vi "Autonomous Independent.vi"() -> ()   [LabVIEW 2015]
doc: "This VI is called when autonomous begins, and will automatically be terminated when autonomous ends. You can carry out timed or sensor driven robot movement independently without needing to return to the caller."
uses:
  <vilib>/Rock Robotics/WPI/DriverStation/WPI_DriverStationMatch Info.ctl
  <vilib>/Rock Robotics/WPI/Utilities/WPI_GetSetVariantRefNum.vi
  <vilib>/Rock Robotics/Network Tables/NT Write Numeric Array.vi
  <vilib>/Rock Robotics/Network Tables/NT Read String.vi
  <vilib>/Rock Robotics/WPI/Solenoid/Deprecated/WPI_SolenoidSetBool.vi
  <vilib>/Rock Robotics/WPI/RobotDrive/WPI_RobotDriveArcadeDrive_Standard(NoSaturation).vi
  Global 1.vi
  Global 2.vi
  <vilib>/functionblocks/Counter/Pulse Timer/Pulse Timer.vi
  <vilib>/functionblocks/Counter/Timer On Delay/Timer On Delay.vi
  <vilib>/Rock Robotics/Network Tables/NT Write Boolean.vi
  <vilib>/functionblocks/FB Core/FB Core.xnode
  <vilib>/Rock Robotics/WPI/SafetyOutput/WPI_SafetyOutputConfigMenu.ctl
  <vilib>/functionblocks/NI_FunctionBlock Libraries.lvlib
panel:
  out "Actual Arm Angle":dbl
  out "Arm Speed":dbl
  out "Arm Request":dbl
  out "Vert Gyro Angle":dbl
  out "Horz Gyro Angle":dbl
  out "Position":string
  out "Defense":string
  out "Right Distance":dbl
  out "Left Distance":dbl
  in  "Match Info":T1={"Autonomous Elapsed Seconds"=0.0, "TeleOp Elapsed Seconds"=0.0, "Disabled Elapsed Seconds"=0.0, "Visited Autonomous"=FALSE, "Visited TeleOp"=FALSE, "Visited Disabled"=FALSE, "Autonomous Settings"={"Autonomous Style"=enum."Independent", "VI Refnum"=refnum}}
  out "Current Movement, for debugging":T2 {"Y Joystick Value" scale=1.0..-1.0; "X Joystick Value" scale=-1.0..1.0}
  in  "Array of robot movements":T3(array[cluster])=[{"X Joystick Value"=0.39393939393939403, "Y Joystick Value"=0.0, "Delay (sec)"=1.0, "Movement Name"="turn"}, {"X Joystick Value"=-0.3737373737373737, "Y Joystick Value"=0.0, "Delay (sec)"=1.0, "Movement Name"="turn back"}] {"Y Joystick Value" scale=1.0..-1.0; "X Joystick Value" scale=-1.0..1.0}
  # "Be sure to right-click and choose Data Operations>>Make Current Value default if you want to save the array values with the VI"
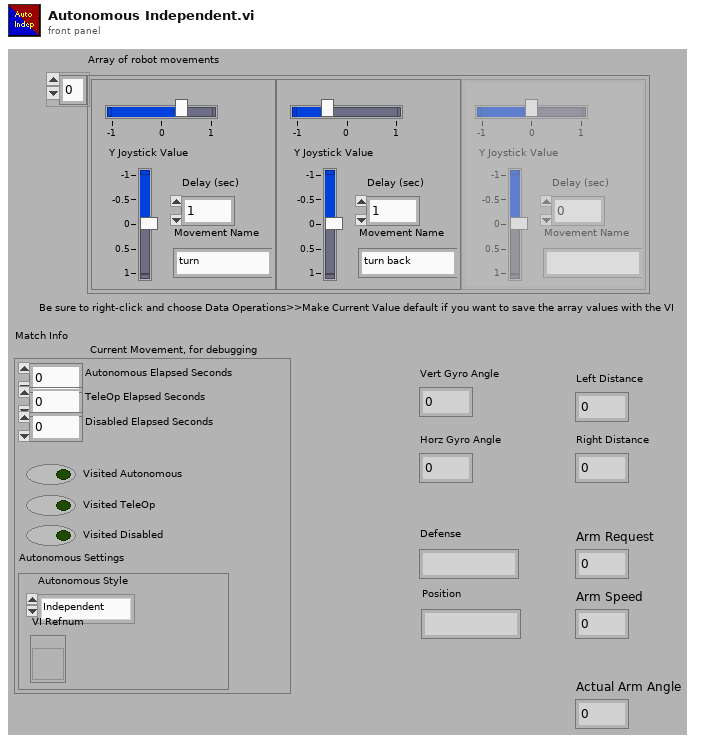
[diagram p1: front panel]
types:
  T1 = typedef "WPI_DriverStationMatch Info.ctl" = cluster{"Autonomous Elapsed Seconds":dbl, "TeleOp Elapsed Seconds":dbl, "Disabled Elapsed Seconds":dbl, "Visited Autonomous":bool, "Visited TeleOp":bool, "Visited Disabled":bool, "Autonomous Settings":cluster{"Autonomous Style":enum16{"Iterative", "Independent"}, "VI Refnum":refnum<vi>}}
  T2 = cluster{"X Joystick Value":dbl, "Y Joystick Value":dbl, "Delay (sec)":dbl, "Movement Name":string}
  T3 = cluster{"X Joystick Value":dbl, "Y Joystick Value":dbl, "Delay (sec)":dbl, "Movement Name":string}[]
  T4 = typedef "WPI_GyroDevRef.ctl" = cluster{"DevStatus":errorcluster, "Analog Channel":T5, "Offset":dbl, "Gain (VoltsPerDegree/Second)":dbl, "Gyro Type":enum16{"Analog", "XRS450"}, "Handle":i32, "SPI Bus":T6, "Device Found":bool, "Sample Rate":dbl, "Calibrate On Open":bool}
  T5 = typedef "FPGA_AIChannel.ctl" = enum8{"AI 0", "AI 1", "AI 2", "AI 3", "AI MXP 0", "AI MXP 1", "AI MXP 2", "AI MXP 3", "Invalid"}
  T6 = typedef "spi_bus.ctl" = enum16{"SPI On-Board, CS0", "SPI On-Board, CS1", "SPI On-Board, CS2", "SPI On-Board, CS3", "SPI MXP", "Invalid"}
  T7 = typedef "WPI_EncoderDevRef.ctl" = cluster{"DevStatus":errorcluster, "EncoderIndex":T8, "CounterIndex":T9, "DistancePerCount":dbl, "Decoding Type":T10}
  T8 = typedef "FPGA_EncoderIdx.ctl" = enum8{"Enc 0", "Enc 1", "Enc 2", "Enc 3", "Enc 4", "Enc 5", "Enc 6", "Enc 7", "Invalid"}
  T9 = typedef "FPGA_CounterCtrSystemIndex.ctl" = enum8{"Ctr 0", "Ctr 1", "Ctr 2", "Ctr 3", "Ctr 4", "Ctr 5", "Ctr 6", "Ctr 7", "Invalid"}
  T10 = typedef "WPI_EncoderType.ctl" = enum16{"1x", "2x", "4x"}
  T11 = typedef "WPI_JoystickDevRef.ctl" = cluster{"Device":T12}
  T12 = typedef "WPI_JoystickDeviceEnum.ctl" = enum16{"USB 0", "USB 1", "USB 2", "USB 3", "USB 4", "USB 5"}
  T13 = typedef "WPI_PotentiometerDevRef.ctl" = cluster{"DevStatus":errorcluster, "Analog Channel":T5, "Invert Output":bool}
  T14 = typedef "WPI_SolenoidDevRef.ctl" = cluster{"DevStatus":errorcluster, "Pneumatics Control Module":u8, "Forward Solenoid Channel":T15, "Reverse Solenoid Channel":T15}
  T15 = typedef "WPI_SolenoidChannel.ctl" = enum8{"Solenoid 0", "Solenoid 1", "Solenoid 2", "Solenoid 3", "Solenoid 4", "Solenoid 5", "Solenoid 6", "Solenoid 7", "Invalid"}
  T16 = typedef "WPI_RobotDriveDevRef.ctl" = cluster{"DevStatus":errorcluster, "Motors[]":T17[], "Square Inputs":bool, "Max Output":dbl}
  T17 = typedef "WPI_MotorControlDeviceRef.ctl" = cluster{"DeviceStatus":errorcluster, "Type":T18, "PWM":cluster{"PWM Channel":T19, "DeadBand":T20}, "CAN":cluster{"Device Number":u8, "Control Mode":T21, "Semaphore":T22, "Max Vout":dbl, "TalonSRX Control Mode":T23}, "Invert":bool}
  T18 = typedef "WPI_MotorControlType.ctl" = enum16{"PWM", "CAN", "CANTalonSRX"}
  T19 = typedef "FPGA_DIOPWMChannel.ctl" = enum8{"PWM 0", "PWM 1", "PWM 2", "PWM 3", "PWM 4", "PWM 5", "PWM 6", "PWM 7", "PWM 8", "PWM 9", "PWM MXP 0", "PWM MXP 1", "PWM MXP 2", "PWM MXP 3", "PWM MXP 4", "PWM MXP 5", "PWM MXP 6", "PWM MXP 7", "PWM MXP 8", "PWM MXP 9", "Invalid"}
  T20 = typedef "WPI_PWMDeadband.ctl" = cluster{"Name":string, "maxPositivePwm":i32, "minPositivePwm":i32, "centerPwm":i32, "maxNegativePwm":i32, "minNegativePwm":i32, "angularRange":u16}
  T21 = typedef "WPI_CANJaguar_ControlMode.ctl" = enum8{"Percent VBus", "Current", "Speed", "Position", "Voltage"}
  T22 = typedef "Semaphore RefNum" = refnum<k1>
  T23 = typedef "WPI_CANTalonSRX_APIControlMode.ctl" = enum8{"Percent VBus", "Speed", "Position", "Slave", "Unchanged / Invalid", "Voltage Compensation", "Current", "Motion Profile"}
  T24 = cluster{"X-Axis":dbl, "Y-Axis":dbl, "Z-Axis":dbl}
  T25 = typedef "WPI_SafetyOutputConfigMenu.ctl" = enum16{"Enable", "Disable"}
  T26 = typedef "WPI_AccelerometerDevRef.ctl" = cluster{"DevStatus":errorcluster, "Scaling":T27, "Analog Channels":T28, "I2C Bus":T29, "SPI Bus":T6, "Accel Range":T30, "ADXL Axes":T31, "Handle":i32, "Device Address":u8, "Accel Type":enum16{"Analog", "ADXL345 I2C", "ADXL345 SPI", "Internal", "ADXL362 SPI"}}
  T27 = typedef "WPI_AccelerometerScaling.ctl" = cluster{"Gain (VoltsPerG)":dbl, "Center Voltage":dbl}
  T28 = typedef "WPI_AccelerometerAnalogChannels.ctl" = cluster{"X-Axis":T5, "Y-Axis":T5, "Z-Axis":T5}
  T29 = typedef "i2c_bus.ctl" = enum16{"I2C On-Board", "I2C MXP", "Invalid"}
  T30 = typedef "ADXL345 Range.ctl" = u8
  T31 = typedef "WPI_AccelerometerADXL345 Axes.ctl" = cluster{"X-Axis":bool, "Y-Axis":bool, "Z-Axis":bool}
  T32 = typedef "WPI_RelayDevRef.ctl" = cluster{"DevStatus":errorcluster, "Relay Channel":T33, "Relay Direction":T34}
  T33 = typedef "FPGA_DIORelayChannel.ctl" = enum8{"Relay 0", "Relay 1", "Relay 2", "Relay 3", "Invalid"}
  T34 = typedef "WPI_RelayDirection.ctl" = enum16{"Both directions", "Forward only", "Reverse only"}
  T35 = typedef "WPI_ServoDeviceRef.ctl" = cluster{"DeviceStatus":errorcluster, "PWM Channel":T19, "DeadBand":T20}
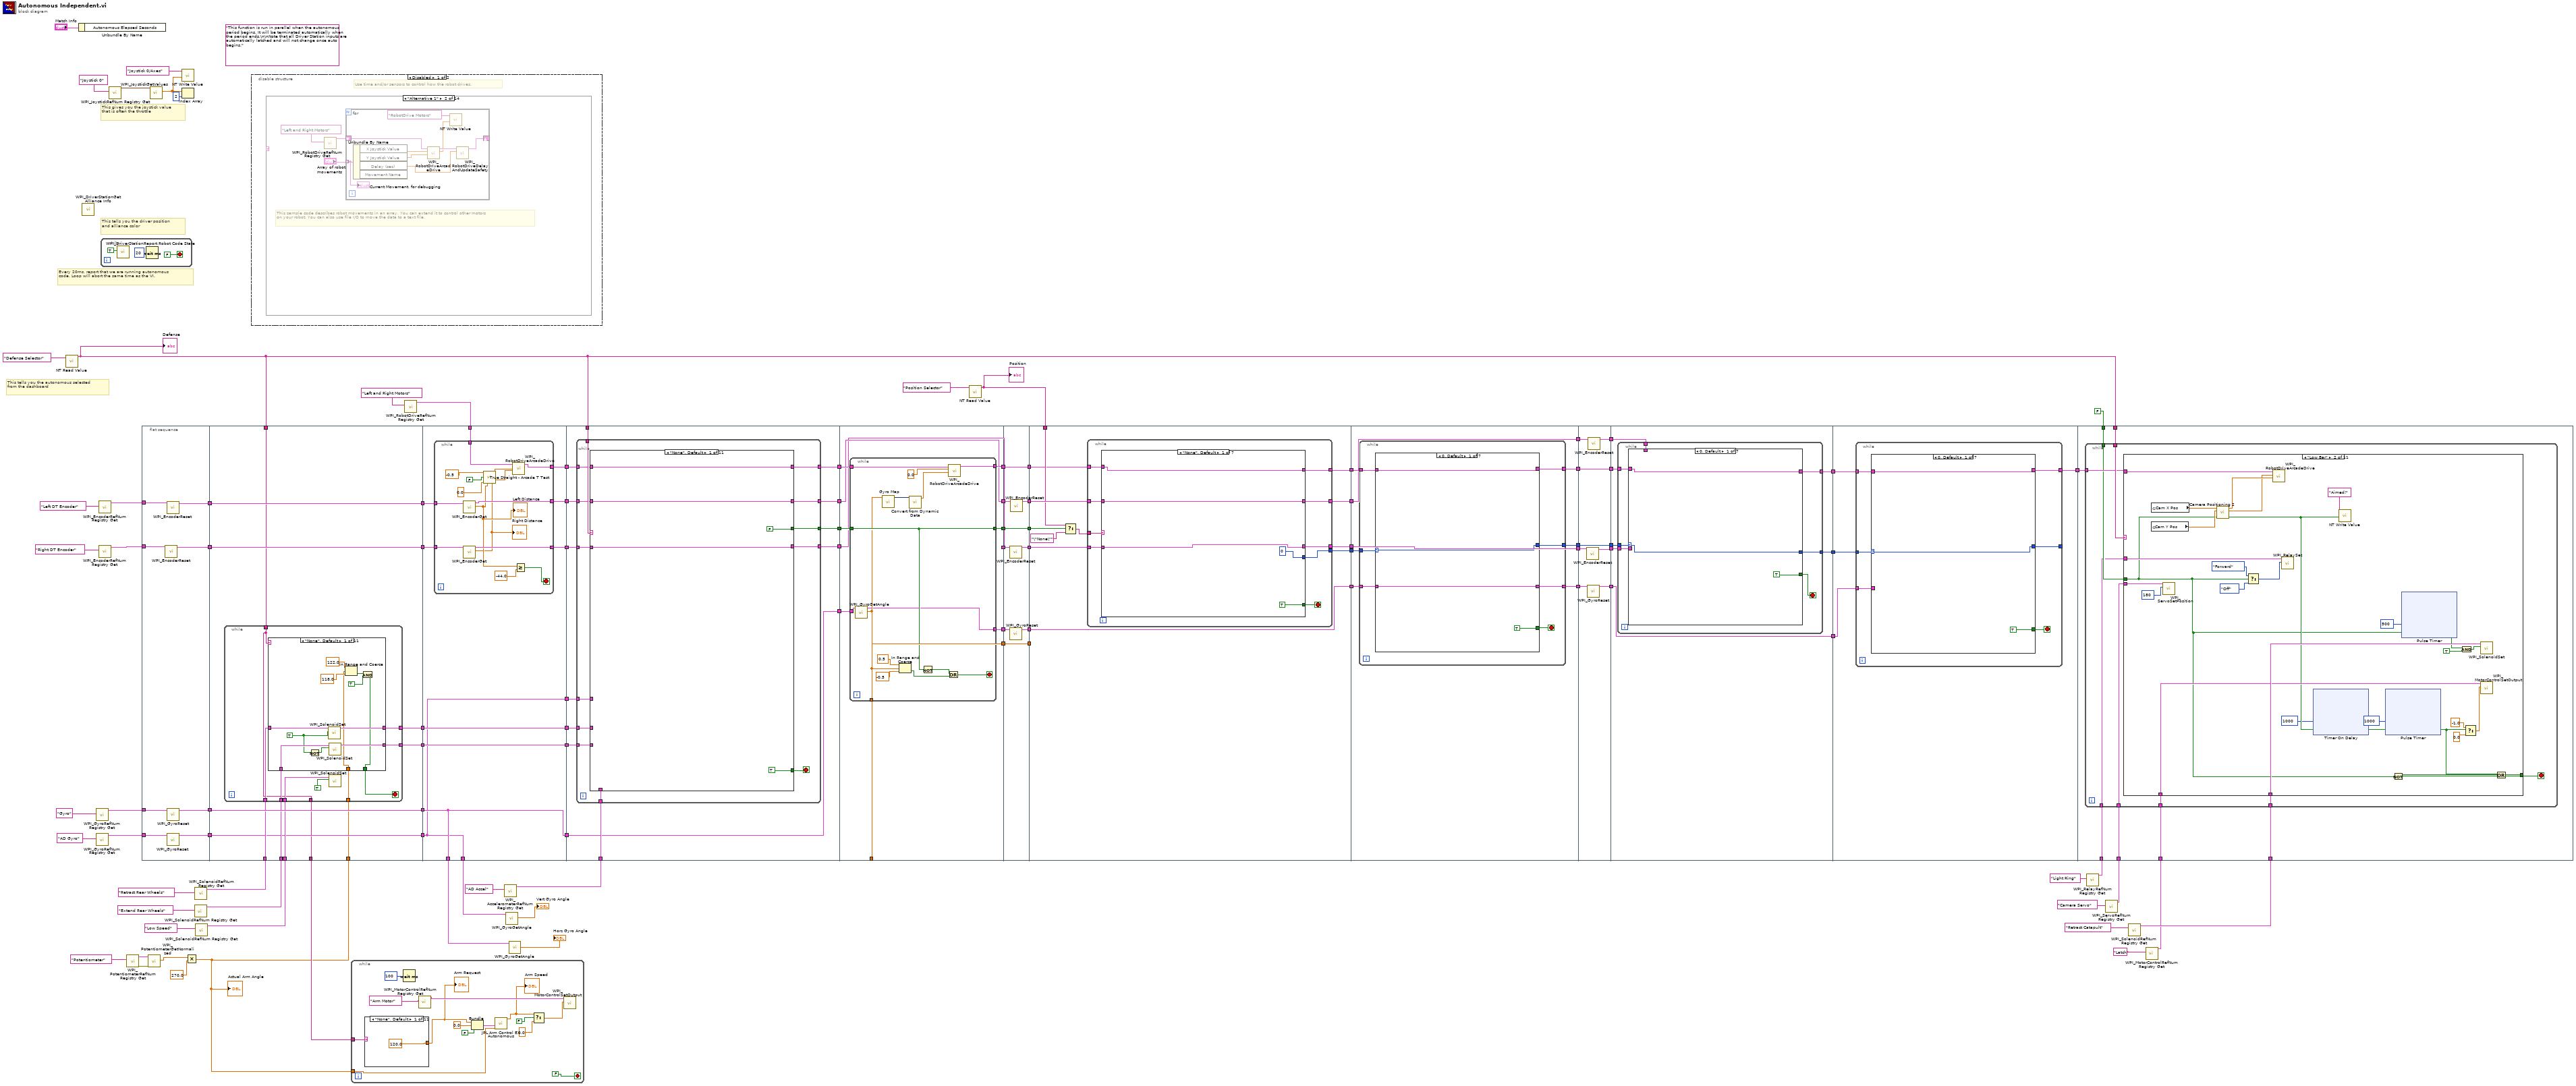
[diagram p0: block diagram]
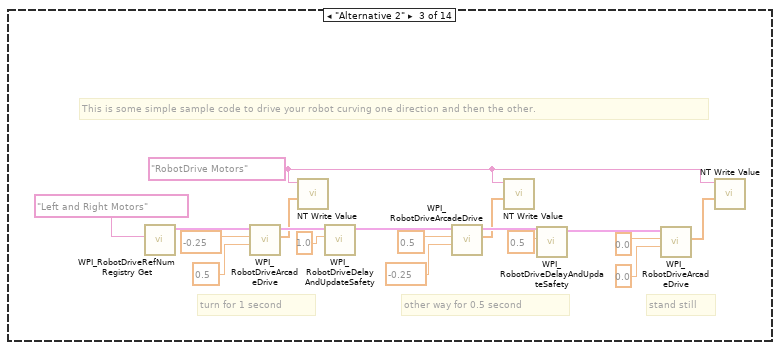
[diagram p3: hidden frame]
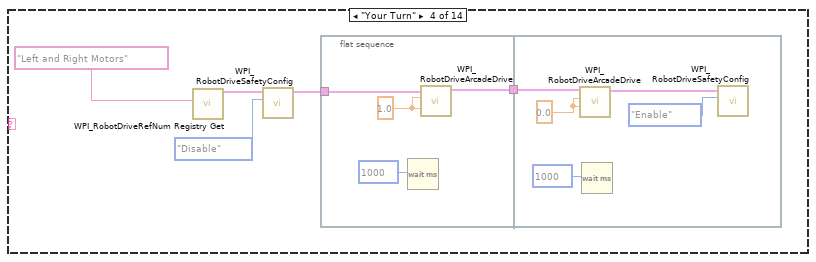
[diagram p4: hidden frame]
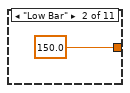
[diagram p16: hidden frame]
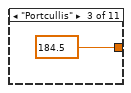
[diagram p17: hidden frame]
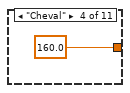
[diagram p18: hidden frame]
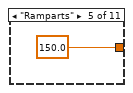
[diagram p19: hidden frame]
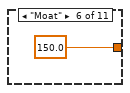
[diagram p20: hidden frame]
diagram:
  (unwired) "This function is run in parallel when the autonomous period begins. It will be terminated automatically when the period ends.\n\nNote that all Driver Station inputs are automatically latched and will not change once auto begins."
  # "This tells you the autonomous selected\nfrom the dashboard"
  # "Every 20ms, report that we are running autonomous\ncode. Loop will abort the same time as the VI."
  # "This gives you the joystick value\nthat is often the throttle"
  # "This tells you the driver position\nand alliance color"
  n1 = call-poly <vilib>:"NT Read Value.vi"("Name"="Defense Selector") -> ("String"=w13:string)  [unwired: 9 in, 1 out]
  "Defense" <- w13
  n2 = Unbundle By Name("Match Info") -> ()  [unwired: 1 out]
  n3 = call <vilib>:"WPI_DriverStationGet Alliance Info.vi"() -> ()  [unwired: 12 out]
  n4 = call <vilib>:"WPI_GyroRefNum Registry Get.vi"("refnum name"="Gyro") -> ("GyroDevRef"=w80:T4)  [unwired: 9 in, 1 out]
  n5 = call <vilib>:"WPI_GyroRefNum Registry Get.vi"("refnum name"="AD Gyro") -> ("GyroDevRef"=w54:T4)  [unwired: 9 in, 1 out]
  n6 = call <vilib>:"WPI_EncoderRefNum Registry Get.vi"("refnum name"="Left DT Encoder") -> ("EncoderDevRef"=w84:T7)  [unwired: 9 in, 1 out]
  n7 = call <vilib>:"WPI_EncoderRefNum Registry Get.vi"("refnum name"="Right DT Encoder") -> ("EncoderDevRef"=w83:T7)  [unwired: 9 in, 1 out]
  n8 = while {
    stop <- FALSE stop-if-true
    n9 = call <vilib>:"WPI_DriverStationReport Robot Code State.vi"("Autonomous"=TRUE) -> ()  [unwired: 10 in, 1 out]
    n10 = Wait (ms)(milliseconds to wait=u32 20) -> ()  [unwired: 1 out]
  }
  n11 = call <vilib>:"WPI_JoystickRefNum Registry Get.vi"("refnum name"="Joystick 0") -> ("JoystickDevRef"=w100:T11)  [unwired: 1 in, 9 out]
  n12 = call <vilib>:"WPI_PotentiometerRefNum Registry Get.vi"("refnum name"="Potentiometer") -> ("error out"=w45:errorcluster, "PotDevRef"=w44:T13)  [unwired: 9 in]
  n13 = flat-sequence {
    tunnel: w84 -> [w112]
    tunnel: [w111] -> w72
    tunnel: [w110] -> w70
    tunnel: w83 -> [w109]
    tunnel: w80 -> [w108]
    tunnel: [w107] -> w68
    tunnel: w54 -> [w106]
    tunnel: [w105] -> w52
    tunnel: w72 -> [w124]
    tunnel: [w124] -> w71
    tunnel: w70 -> [w123]
    tunnel: [w123] -> w69
    tunnel: w68 -> [w122]
    tunnel: [w122] -> w67
    tunnel: w63 -> [w121]
    tunnel: w61 -> [w120]
    tunnel: w60 -> [w119]
    tunnel: w13 -> [w118]
    tunnel: [w117] -> w58
    tunnel: [w116] -> w56
    tunnel: [w115] -> w53
    tunnel: w52 -> [w115]
    tunnel: w1 -> [w114]
    tunnel: [w113] -> w43
    tunnel: w71 -> [w255]
    tunnel: w69 -> [w254]
    tunnel: w79 -> [w253]
    tunnel: [w252] -> w94
    tunnel: [w251] -> w93
    tunnel: [w250] -> w92
    tunnel: w67 -> [w247]
    tunnel: [w247] -> w74
    tunnel: [w249] -> w59
    tunnel: w58 -> [w249]
    tunnel: [w248] -> w57
    tunnel: w56 -> [w248]
    tunnel: w53 -> [w246]
    tunnel: [w246] -> w51
    tunnel: [w247] -> w41
    tunnel: [w246] -> w39
    tunnel: w13 -> [w283]
    tunnel: w94 -> [w282]
    tunnel: w93 -> [w281]
    tunnel: w92 -> [w280]
    tunnel: w78 -> [w279]
    tunnel: [w278] -> w91
    tunnel: [w277] -> w90
    tunnel: [w276] -> w89
    tunnel: [w275] -> w88
    tunnel: w59 -> [w274]
    tunnel: w57 -> [w273]
    tunnel: [w272] -> w42
    tunnel: w41 -> [w272]
    tunnel: w39 -> [w271]
    tunnel: w91 -> [w558]
    tunnel: [w557] -> w27
    tunnel: w90 -> [w554]
    tunnel: [w554] -> w29
    tunnel: w89 -> [w553]
    tunnel: [w553] -> w31
    tunnel: w88 -> [w556]
    tunnel: [w555] -> w33
    tunnel: [w552] -> _
    tunnel: [w552] -> w35
    tunnel: w42 -> [w551]
    tunnel: [w550] -> w25
    tunnel: w35 -> [w581]
    tunnel: [w581] -> w34
    tunnel: w33 -> [w580]
    tunnel: [w580] -> w32
    tunnel: w31 -> [w576]
    tunnel: [w575] -> w30
    tunnel: w29 -> [w574]
    tunnel: [w573] -> w28
    tunnel: w27 -> [w579]
    tunnel: [w579] -> w26
    tunnel: w25 -> [w578]
    tunnel: [w577] -> w24
    tunnel: w75 -> [w591]
    tunnel: [w588] -> w49
    tunnel: [w587] -> w48
    tunnel: [w586] -> w47
    tunnel: [w585] -> w46
    tunnel: w34 -> [_]
    tunnel: w32 -> [w583]
    tunnel: w30 -> [w592]
    tunnel: w28 -> [w593]
    tunnel: w26 -> [w584]
    tunnel: [w582] -> w40
    tunnel: w24 -> [w582]
    tunnel: w49 -> [w711]
    tunnel: w48 -> [w710]
    tunnel: [w709] -> w23
    tunnel: [w708] -> w21
    tunnel: [w707] -> w19
    tunnel: w47 -> [w707]
    tunnel: [w706] -> w17
    tunnel: w46 -> [w706]
    tunnel: w40 -> [w705]
    tunnel: [w704] -> w15
    tunnel: w23 -> [w794]
    tunnel: [w794] -> w22
    tunnel: w21 -> [w793]
    tunnel: [w793] -> w20
    tunnel: w19 -> [w790]
    tunnel: [w789] -> w18
    tunnel: w17 -> [w792]
    tunnel: [w791] -> w16
    tunnel: w15 -> [w788]
    tunnel: [w787] -> w14
    tunnel: w22 -> [w801]
    tunnel: w20 -> [w800]
    tunnel: w18 -> [w799]
    tunnel: w16 -> [w798]
    tunnel: [w797] -> w38
    tunnel: [w796] -> w37
    tunnel: [w795] -> w36
    tunnel: w14 -> [w795]
    tunnel: w36 -> [w875]
    tunnel: w37 -> [w876]
    tunnel: w38 -> [w877]
    tunnel: [w874] -> w10
    tunnel: w13 -> [w971]
    tunnel: w10 -> [w970]
    tunnel: w9 -> [w969]
    tunnel: FALSE -> [w968]
    tunnel: w7 -> [w967]
    tunnel: w5 -> [w966]
    tunnel: w4 -> [w965]
    frame #0 {
      n14 = call <vilib>:"WPI_EncoderReset.vi"("EncoderDevRef"=w109) -> ("EncoderDevRef"=w110:T7)  [unwired: 9 in, 1 out]
      n15 = call <vilib>:"WPI_EncoderReset.vi"("EncoderDevRef"=w112) -> ("EncoderDevRef"=w111:T7)  [unwired: 9 in, 1 out]
      n16 = call <vilib>:"WPI_GyroReset.vi"("GyroDevRef"=w106) -> ("GyroDevRef"=w105:T4)  [unwired: 9 in, 1 out]
      n17 = call <vilib>:"WPI_GyroReset.vi"("GyroDevRef"=w108) -> ("GyroDevRef"=w107:T4)  [unwired: 9 in, 1 out]
    }
    frame #1 {
      n18 = while {
        tunnel: w121 -> [w133]
        tunnel: w120 -> [w131]
        tunnel: w119 -> [w129]
        tunnel: w118 -> [w125]
        tunnel: [w128] -> w117
        tunnel: [w127] -> w116
        tunnel: w114 -> [w126]
        tunnel: [w125] -> w113
        stop <- w130 stop-if-true
        n19 = case shown="\"None\", Default" w125 {
          tunnel: w131 -> [w145 w155 w165 w175 w185 w195 w205 w215 w225 w235 w245]
          tunnel: [w136 w152 w162 w172 w182 w192 w202 w212 w222 w232 w242] -> w130
          tunnel: w129 -> [w143 w151 w161 w171 w181 w191 w201 w211 w221 w231 w241]
          tunnel: [w142 w148 w158 w168 w178 w188 w198 w208 w218 w228 w238] -> w128
          tunnel: [w141 w147 w157 w167 w177 w187 w197 w207 w217 w227 w237] -> w127
          tunnel: w126 -> [w134 w146 w156 w166 w176 w186 w196 w206 w216 w226 w236]
          frame "None", Default {
            w137 = TRUE
            n20 = Not(x=w137) -> (.not. x?=w144:bool)
            n21 = call-poly <vilib>:"WPI_SolenoidSet.vi"("Value"=w137, "SolenoidDevRef"=w143) -> ("SolenoidDevRef"=w142:T14)  [unwired: 8 in, 1 out]
            n22 = call-poly <vilib>:"WPI_SolenoidSet.vi"("Value"=w144, "SolenoidDevRef"=w145) -> ("SolenoidDevRef"=w141:T14)  [unwired: 8 in, 1 out]
            n23 = In Range and Coerce(upper limit=122.0, x=w134, lower limit=118.0) -> (In Range?=w138:bool)  [unwired: 1 out]
            n24 = And(x=w138, y=TRUE) -> (x .and. y?=w136:bool)
          }
          frame "Low Bar" {
            w153 = TRUE
            n25 = Not(x=w153) -> (.not. x?=w154:bool)
            n26 = call-poly <vilib>:"WPI_SolenoidSet.vi"("Value"=w153, "SolenoidDevRef"=w151) -> ("SolenoidDevRef"=w148:T14)  [unwired: 8 in, 1 out]
            n27 = call-poly <vilib>:"WPI_SolenoidSet.vi"("Value"=w154, "SolenoidDevRef"=w155) -> ("SolenoidDevRef"=w147:T14)  [unwired: 8 in, 1 out]
            n28 = In Range and Coerce(upper limit=152.0, x=w146, lower limit=148.0) -> (In Range?=w152:bool)  [unwired: 1 out]
          }
          frame "Portcullis" {
            w163 = TRUE
            n29 = Not(x=w163) -> (.not. x?=w164:bool)
            n30 = call-poly <vilib>:"WPI_SolenoidSet.vi"("Value"=w163, "SolenoidDevRef"=w161) -> ("SolenoidDevRef"=w158:T14)  [unwired: 8 in, 1 out]
            n31 = call-poly <vilib>:"WPI_SolenoidSet.vi"("Value"=w164, "SolenoidDevRef"=w165) -> ("SolenoidDevRef"=w157:T14)  [unwired: 8 in, 1 out]
            n32 = In Range and Coerce(upper limit=186.0, x=w156, lower limit=182.0) -> (In Range?=w162:bool)  [unwired: 1 out]
          }
          frame "Cheval" {
            w173 = TRUE
            n33 = Not(x=w173) -> (.not. x?=w174:bool)
            n34 = call-poly <vilib>:"WPI_SolenoidSet.vi"("Value"=w173, "SolenoidDevRef"=w171) -> ("SolenoidDevRef"=w168:T14)  [unwired: 8 in, 1 out]
            n35 = call-poly <vilib>:"WPI_SolenoidSet.vi"("Value"=w174, "SolenoidDevRef"=w175) -> ("SolenoidDevRef"=w167:T14)  [unwired: 8 in, 1 out]
            n36 = In Range and Coerce(upper limit=162.0, x=w166, lower limit=158.0) -> (In Range?=w172:bool)  [unwired: 1 out]
          }
          frame "Ramparts" {
            w183 = FALSE
            n37 = Not(x=w183) -> (.not. x?=w184:bool)
            n38 = call-poly <vilib>:"WPI_SolenoidSet.vi"("Value"=w183, "SolenoidDevRef"=w181) -> ("SolenoidDevRef"=w178:T14)  [unwired: 8 in, 1 out]
            n39 = call-poly <vilib>:"WPI_SolenoidSet.vi"("Value"=w184, "SolenoidDevRef"=w185) -> ("SolenoidDevRef"=w177:T14)  [unwired: 8 in, 1 out]
            n40 = In Range and Coerce(upper limit=152.0, x=w176, lower limit=148.0) -> (In Range?=w182:bool)  [unwired: 1 out]
          }
          frame "Moat" {
            w193 = FALSE
            n41 = Not(x=w193) -> (.not. x?=w194:bool)
            n42 = call-poly <vilib>:"WPI_SolenoidSet.vi"("Value"=w193, "SolenoidDevRef"=w191) -> ("SolenoidDevRef"=w188:T14)  [unwired: 8 in, 1 out]
            n43 = call-poly <vilib>:"WPI_SolenoidSet.vi"("Value"=w194, "SolenoidDevRef"=w195) -> ("SolenoidDevRef"=w187:T14)  [unwired: 8 in, 1 out]
            n44 = In Range and Coerce(upper limit=152.0, x=w186, lower limit=148.0) -> (In Range?=w192:bool)  [unwired: 1 out]
          }
          frame "Drawbridge" {
            w203 = TRUE
            n45 = Not(x=w203) -> (.not. x?=w204:bool)
            n46 = call-poly <vilib>:"WPI_SolenoidSet.vi"("Value"=w203, "SolenoidDevRef"=w201) -> ("SolenoidDevRef"=w198:T14)  [unwired: 8 in, 1 out]
            n47 = call-poly <vilib>:"WPI_SolenoidSet.vi"("Value"=w204, "SolenoidDevRef"=w205) -> ("SolenoidDevRef"=w197:T14)  [unwired: 8 in, 1 out]
            n48 = In Range and Coerce(upper limit=122.0, x=w196, lower limit=118.0) -> (In Range?=w202:bool)  [unwired: 1 out]
          }
          frame "Sally Port" {
            w213 = TRUE
            n49 = Not(x=w213) -> (.not. x?=w214:bool)
            n50 = call-poly <vilib>:"WPI_SolenoidSet.vi"("Value"=w213, "SolenoidDevRef"=w211) -> ("SolenoidDevRef"=w208:T14)  [unwired: 8 in, 1 out]
            n51 = call-poly <vilib>:"WPI_SolenoidSet.vi"("Value"=w214, "SolenoidDevRef"=w215) -> ("SolenoidDevRef"=w207:T14)  [unwired: 8 in, 1 out]
            n52 = In Range and Coerce(upper limit=162.0, x=w206, lower limit=158.0) -> (In Range?=w212:bool)  [unwired: 1 out]
          }
          frame "Rock Wall" {
            w223 = FALSE
            n53 = Not(x=w223) -> (.not. x?=w224:bool)
            n54 = call-poly <vilib>:"WPI_SolenoidSet.vi"("Value"=w223, "SolenoidDevRef"=w221) -> ("SolenoidDevRef"=w218:T14)  [unwired: 8 in, 1 out]
            n55 = call-poly <vilib>:"WPI_SolenoidSet.vi"("Value"=w224, "SolenoidDevRef"=w225) -> ("SolenoidDevRef"=w217:T14)  [unwired: 8 in, 1 out]
            n56 = In Range and Coerce(upper limit=152.0, x=w216, lower limit=148.0) -> (In Range?=w222:bool)  [unwired: 1 out]
          }
          frame "Rough Terrain" {
            w233 = FALSE
            n57 = Not(x=w233) -> (.not. x?=w234:bool)
            n58 = call-poly <vilib>:"WPI_SolenoidSet.vi"("Value"=w233, "SolenoidDevRef"=w231) -> ("SolenoidDevRef"=w228:T14)  [unwired: 8 in, 1 out]
            n59 = call-poly <vilib>:"WPI_SolenoidSet.vi"("Value"=w234, "SolenoidDevRef"=w235) -> ("SolenoidDevRef"=w227:T14)  [unwired: 8 in, 1 out]
            n60 = In Range and Coerce(upper limit=152.0, x=w226, lower limit=148.0) -> (In Range?=w232:bool)  [unwired: 1 out]
          }
          frame "Test" {
            w243 = FALSE
            n61 = Not(x=w243) -> (.not. x?=w244:bool)
            n62 = call-poly <vilib>:"WPI_SolenoidSet.vi"("Value"=w243, "SolenoidDevRef"=w241) -> ("SolenoidDevRef"=w238:T14)  [unwired: 8 in, 1 out]
            n63 = call-poly <vilib>:"WPI_SolenoidSet.vi"("Value"=w244, "SolenoidDevRef"=w245) -> ("SolenoidDevRef"=w237:T14)  [unwired: 8 in, 1 out]
            n64 = In Range and Coerce(upper limit=152.0, x=w236, lower limit=148.0) -> (In Range?=w242:bool)  [unwired: 1 out]
          }
        }
        n65 = call-poly <vilib>:"WPI_SolenoidSet.vi"("Value"=TRUE, "SolenoidDevRef"=w133) -> ()  [unwired: 8 in, 2 out]
      }
    }
    frame #2 {
      n66 = while {
        tunnel: w255 -> [w270]
        tunnel: w254 -> [w269]
        tunnel: w253 -> [w268]
        tunnel: [w265] -> w252
        tunnel: [w264] -> w251
        tunnel: [w263] -> w250
        stop <- w267 stop-if-true
        n67 = call <vilib>:"WPI_EncoderGet.vi"("EncoderDevRef"=w270) -> ("Distance"=w260:dbl, "EncoderDevRef"=w264:T7)  [unwired: 5 in, 4 out]
        "Left Distance" <- w260
        n68 = call <vilib>:"WPI_EncoderGet.vi"("EncoderDevRef"=w269) -> ("Distance"=w259:dbl, "EncoderDevRef"=w263:T7)  [unwired: 5 in, 4 out]
        "Right Distance" <- w259
        n69 = call "True Straight - Arcade T Test.vi"("Fwd/Rev Joy"=-0.5, "Bypass"=FALSE, "Left/Right Joy"=0.0, "Left Encoder"=w260, "Right Encoder"=w259) -> ("Fwd/Rev Out"=w258:dbl, "Left/Right Out"=w257:dbl)  [unwired: 8 in, 1 out]
        n70 = call-poly <vilib>:"WPI_RobotDriveArcadeDrive.vi"("Y axis value"=w257, "X axis value"=w258, "RobotDriveDevRef"=w268) -> ("RobotDriveDevRef"=w265:T16)  [unwired: 6 in, 2 out]
        n71 = Greater Or Equal?(x=w260, y=-44.0) -> (x >= y?=w267:bool)
      }
    }
    frame #3 {
      n72 = while {
        tunnel: w283 -> [w296]
        tunnel: w282 -> [w295]
        tunnel: w281 -> [w294]
        tunnel: w280 -> [w293]
        tunnel: w279 -> [w292]
        tunnel: [w290] -> w278
        tunnel: [w289] -> w277
        tunnel: [w288] -> w276
        tunnel: [w287] -> w275
        tunnel: w274 -> [w286]
        tunnel: w273 -> [w285]
        tunnel: w271 -> [w284]
        stop <- w291 stop-if-true
        n73 = case shown="\"None\", Default" w296 {
          tunnel: w295 -> [w298 w339 w343 w346 w387 w425 w427 w432 w473 w511 w549]
          tunnel: w294 -> [w299 w336 w342 w347 w384 w422 w428 w433 w470 w508 w546]
          tunnel: w293 -> [w300 w335 w341 w348 w383 w421 w429 w434 w469 w507 w545]
          tunnel: w292 -> [_ w331 _ _ w379 w417 _ _ w465 w503 w541]
          tunnel: [TRUE w311 TRUE TRUE w359 w397 TRUE TRUE w445 w483 w521] -> w291
          tunnel: [w298 w321 w343 w346 w369 w407 w427 w432 w455 w493 w531] -> w290
          tunnel: [w299 w320 w342 w347 w368 w406 w428 w433 w454 w492 w530] -> w289
          tunnel: [w300 w319 w341 w348 w367 w405 w429 w434 w453 w491 w529] -> w288
          tunnel: [FALSE TRUE FALSE FALSE TRUE TRUE FALSE FALSE TRUE TRUE TRUE] -> w287
          tunnel: w286 -> [_ w313 _ _ w361 w399 _ _ w447 w489 w527]
          tunnel: w285 -> [_ w312 _ _ w360 w398 _ _ w446 w488 w526]
          tunnel: w284 -> [_ w302 _ _ w351 w388 _ _ w437 w474 w512]
          frame "None", Default {
          }
          frame "Low Bar" {
            w314 = TRUE
            n74 = call <vilib>:"WPI_GyroGetAngle.vi"("GyroDevRef"=w302) -> ("Angle"=w303:dbl)  [unwired: 6 in, 4 out]
            n75 = call <vilib>:"WPI_AccelerometerGetAcceleration.vi"("AccelerometerDevRef"=w331) -> ("Accelerations"=w330:T24)  [unwired: 8 in, 2 out]
            n76 = call <vilib>:"WPI_EncoderGet.vi"("EncoderDevRef"=w336) -> ("Distance"=w333:dbl, "EncoderDevRef"=w320:T7)  [unwired: 5 in, 4 out]
            n77 = call <vilib>:"WPI_EncoderGet.vi"("EncoderDevRef"=w335) -> ("Distance"=w334:dbl, "EncoderDevRef"=w319:T7)  [unwired: 5 in, 4 out]
            n78 = Unbundle(w330) -> ("Z-Axis"=w325:dbl)  [unwired: 2 out]
            n79 = In Range and Coerce(upper limit=1.0, x=w303, lower limit=-1.0) -> (In Range?=w309:bool)  [unwired: 1 out]
            n80 = call "True Straight - Arcade T Test.vi"("Fwd/Rev Joy"=-0.5, "Bypass"=FALSE, "Left/Right Joy"=0.0, "Left Encoder"=w333, "Right Encoder"=w334) -> ("Fwd/Rev Out"=w323:dbl, "Left/Right Out"=w322:dbl)  [unwired: 8 in, 1 out]
            n81 = Greater Or Equal?(x=w325, y=0.0) -> (x >= y?=w328:bool)
            n82 = call-poly <vilib>:"WPI_RobotDriveArcadeDrive.vi"("Y axis value"=w322, "X axis value"=w323, "RobotDriveDevRef"=w339) -> ("RobotDriveDevRef"=w321:T16)  [unwired: 6 in, 2 out]
            n83 = Greater Or Equal?(x=w333, y=-130.0) -> (x >= y?=w329:bool)
            n84 = Or(x=w328, y=TRUE) -> (x .or. y?=w305:bool)
            n85 = Or(x=w309, y=TRUE) -> (x .or. y?=w310:bool)
            n86 = Not(x=w314) -> (.not. x?=w315:bool)
            n87 = And(x=w305, y=w310) -> (x .and. y?=w304:bool)
            n88 = And(x=w329, y=w304) -> (x .and. y?=w311:bool)
            n89 = And(x=w311, y=w314) -> (x .and. y?=w317:bool)
            n90 = And(x=w311, y=w315) -> (x .and. y?=w316:bool)
            n91 = call-poly <vilib>:"WPI_SolenoidSet.vi"("Value"=w317, "SolenoidDevRef"=w313) -> ()  [unwired: 8 in, 2 out]
            n92 = call-poly <vilib>:"WPI_SolenoidSet.vi"("Value"=w316, "SolenoidDevRef"=w312) -> ()  [unwired: 8 in, 2 out]
          }
          frame "Portcullis" {
          }
          frame "Cheval" {
          }
          frame "Ramparts" {
            w362 = TRUE
            n93 = call <vilib>:"WPI_GyroGetAngle.vi"("GyroDevRef"=w351) -> ("Angle"=w350:dbl)  [unwired: 6 in, 4 out]
            n94 = call <vilib>:"WPI_AccelerometerGetAcceleration.vi"("AccelerometerDevRef"=w379) -> ("Accelerations"=w378:T24)  [unwired: 8 in, 2 out]
            n95 = call <vilib>:"WPI_EncoderGet.vi"("EncoderDevRef"=w384) -> ("Distance"=w381:dbl, "EncoderDevRef"=w368:T7)  [unwired: 5 in, 4 out]
            n96 = call <vilib>:"WPI_EncoderGet.vi"("EncoderDevRef"=w383) -> ("Distance"=w382:dbl, "EncoderDevRef"=w367:T7)  [unwired: 5 in, 4 out]
            n97 = Unbundle(w378) -> ("Z-Axis"=w373:dbl)  [unwired: 2 out]
            n98 = In Range and Coerce(upper limit=1.0, x=w350, lower limit=-1.0) -> (In Range?=w357:bool)  [unwired: 1 out]
            n99 = call "True Straight - Arcade T Test.vi"("Fwd/Rev Joy"=-0.5, "Bypass"=FALSE, "Left/Right Joy"=0.0, "Left Encoder"=w381, "Right Encoder"=w382) -> ("Fwd/Rev Out"=w371:dbl, "Left/Right Out"=w370:dbl)  [unwired: 8 in, 1 out]
            n100 = Greater Or Equal?(x=w373, y=0.0) -> (x >= y?=w376:bool)
            n101 = call-poly <vilib>:"WPI_RobotDriveArcadeDrive.vi"("Y axis value"=w370, "X axis value"=w371, "RobotDriveDevRef"=w387) -> ("RobotDriveDevRef"=w369:T16)  [unwired: 6 in, 2 out]
            n102 = Greater Or Equal?(x=w381, y=-130.0) -> (x >= y?=w377:bool)
            n103 = Or(x=w376, y=TRUE) -> (x .or. y?=w353:bool)
            n104 = Or(x=w357, y=TRUE) -> (x .or. y?=w358:bool)
            n105 = Not(x=w362) -> (.not. x?=w363:bool)
            n106 = And(x=w353, y=w358) -> (x .and. y?=w352:bool)
            n107 = And(x=w377, y=w352) -> (x .and. y?=w359:bool)
            n108 = And(x=w359, y=w362) -> (x .and. y?=w365:bool)
            n109 = And(x=w359, y=w363) -> (x .and. y?=w364:bool)
            n110 = call-poly <vilib>:"WPI_SolenoidSet.vi"("Value"=w365, "SolenoidDevRef"=w361) -> ()  [unwired: 8 in, 2 out]
            n111 = call-poly <vilib>:"WPI_SolenoidSet.vi"("Value"=w364, "SolenoidDevRef"=w360) -> ()  [unwired: 8 in, 2 out]
          }
          frame "Moat" {
            w400 = TRUE
            n112 = call <vilib>:"WPI_GyroGetAngle.vi"("GyroDevRef"=w388) -> ("Angle"=w389:dbl)  [unwired: 6 in, 4 out]
            n113 = call <vilib>:"WPI_AccelerometerGetAcceleration.vi"("AccelerometerDevRef"=w417) -> ("Accelerations"=w416:T24)  [unwired: 8 in, 2 out]
            n114 = call <vilib>:"WPI_EncoderGet.vi"("EncoderDevRef"=w422) -> ("Distance"=w419:dbl, "EncoderDevRef"=w406:T7)  [unwired: 5 in, 4 out]
            n115 = call <vilib>:"WPI_EncoderGet.vi"("EncoderDevRef"=w421) -> ("Distance"=w420:dbl, "EncoderDevRef"=w405:T7)  [unwired: 5 in, 4 out]
            n116 = Unbundle(w416) -> ("Z-Axis"=w411:dbl)  [unwired: 2 out]
            n117 = In Range and Coerce(upper limit=1.0, x=w389, lower limit=-1.0) -> (In Range?=w395:bool)  [unwired: 1 out]
            n118 = call "True Straight - Arcade T Test.vi"("Fwd/Rev Joy"=-0.5, "Bypass"=FALSE, "Left/Right Joy"=0.0, "Left Encoder"=w419, "Right Encoder"=w420) -> ("Fwd/Rev Out"=w409:dbl, "Left/Right Out"=w408:dbl)  [unwired: 8 in, 1 out]
            n119 = Greater Or Equal?(x=w411, y=0.0) -> (x >= y?=w414:bool)
            n120 = call-poly <vilib>:"WPI_RobotDriveArcadeDrive.vi"("Y axis value"=w408, "X axis value"=w409, "RobotDriveDevRef"=w425) -> ("RobotDriveDevRef"=w407:T16)  [unwired: 6 in, 2 out]
            n121 = Or(x=w395, y=TRUE) -> (x .or. y?=w396:bool)
            n122 = Or(x=w414, y=TRUE) -> (x .or. y?=w391:bool)
            n123 = Greater Or Equal?(x=w419, y=-130.0) -> (x >= y?=w415:bool)
            n124 = Not(x=w400) -> (.not. x?=w401:bool)
            n125 = And(x=w391, y=w396) -> (x .and. y?=w390:bool)
            n126 = And(x=w415, y=w390) -> (x .and. y?=w397:bool)
            n127 = And(x=w397, y=w400) -> (x .and. y?=w403:bool)
            n128 = And(x=w397, y=w401) -> (x .and. y?=w402:bool)
            n129 = call-poly <vilib>:"WPI_SolenoidSet.vi"("Value"=w403, "SolenoidDevRef"=w399) -> ()  [unwired: 8 in, 2 out]
            n130 = call-poly <vilib>:"WPI_SolenoidSet.vi"("Value"=w402, "SolenoidDevRef"=w398) -> ()  [unwired: 8 in, 2 out]
          }
          frame "Drawbridge" {
          }
          frame "Sally Port" {
          }
          frame "Rock Wall" {
            w448 = TRUE
            n131 = call <vilib>:"WPI_GyroGetAngle.vi"("GyroDevRef"=w437) -> ("Angle"=w436:dbl)  [unwired: 6 in, 4 out]
            n132 = call <vilib>:"WPI_AccelerometerGetAcceleration.vi"("AccelerometerDevRef"=w465) -> ("Accelerations"=w464:T24)  [unwired: 8 in, 2 out]
            n133 = call <vilib>:"WPI_EncoderGet.vi"("EncoderDevRef"=w470) -> ("Distance"=w467:dbl, "EncoderDevRef"=w454:T7)  [unwired: 5 in, 4 out]
            n134 = call <vilib>:"WPI_EncoderGet.vi"("EncoderDevRef"=w469) -> ("Distance"=w468:dbl, "EncoderDevRef"=w453:T7)  [unwired: 5 in, 4 out]
            n135 = In Range and Coerce(upper limit=1.0, x=w436, lower limit=-1.0) -> (In Range?=w443:bool)  [unwired: 1 out]
            n136 = Unbundle(w464) -> ("Z-Axis"=w459:dbl)  [unwired: 2 out]
            n137 = call "True Straight - Arcade T Test.vi"("Fwd/Rev Joy"=-0.5, "Bypass"=FALSE, "Left/Right Joy"=0.0, "Left Encoder"=w467, "Right Encoder"=w468) -> ("Fwd/Rev Out"=w457:dbl, "Left/Right Out"=w456:dbl)  [unwired: 8 in, 1 out]
            n138 = Greater Or Equal?(x=w459, y=0.0) -> (x >= y?=w462:bool)
            n139 = call-poly <vilib>:"WPI_RobotDriveArcadeDrive.vi"("Y axis value"=w456, "X axis value"=w457, "RobotDriveDevRef"=w473) -> ("RobotDriveDevRef"=w455:T16)  [unwired: 6 in, 2 out]
            n140 = Or(x=w443, y=TRUE) -> (x .or. y?=w444:bool)
            n141 = Or(x=w462, y=TRUE) -> (x .or. y?=w439:bool)
            n142 = Greater Or Equal?(x=w467, y=-130.0) -> (x >= y?=w463:bool)
            n143 = Not(x=w448) -> (.not. x?=w449:bool)
            n144 = And(x=w439, y=w444) -> (x .and. y?=w438:bool)
            n145 = And(x=w463, y=w438) -> (x .and. y?=w445:bool)
            n146 = And(x=w445, y=w448) -> (x .and. y?=w451:bool)
            n147 = And(x=w445, y=w449) -> (x .and. y?=w450:bool)
            n148 = call-poly <vilib>:"WPI_SolenoidSet.vi"("Value"=w451, "SolenoidDevRef"=w447) -> ()  [unwired: 8 in, 2 out]
            n149 = call-poly <vilib>:"WPI_SolenoidSet.vi"("Value"=w450, "SolenoidDevRef"=w446) -> ()  [unwired: 8 in, 2 out]
          }
          frame "Rough Terrain" {
            w484 = TRUE
            n150 = call <vilib>:"WPI_GyroGetAngle.vi"("GyroDevRef"=w474) -> ("Angle"=w475:dbl)  [unwired: 6 in, 4 out]
            n151 = call <vilib>:"WPI_AccelerometerGetAcceleration.vi"("AccelerometerDevRef"=w503) -> ("Accelerations"=w502:T24)  [unwired: 8 in, 2 out]
            n152 = call <vilib>:"WPI_EncoderGet.vi"("EncoderDevRef"=w508) -> ("Distance"=w505:dbl, "EncoderDevRef"=w492:T7)  [unwired: 5 in, 4 out]
            n153 = call <vilib>:"WPI_EncoderGet.vi"("EncoderDevRef"=w507) -> ("Distance"=w506:dbl, "EncoderDevRef"=w491:T7)  [unwired: 5 in, 4 out]
            n154 = Unbundle(w502) -> ("Z-Axis"=w497:dbl)  [unwired: 2 out]
            n155 = call "True Straight - Arcade T Test.vi"("Fwd/Rev Joy"=-0.5, "Bypass"=FALSE, "Left/Right Joy"=0.0, "Left Encoder"=w505, "Right Encoder"=w506) -> ("Fwd/Rev Out"=w495:dbl, "Left/Right Out"=w494:dbl)  [unwired: 8 in, 1 out]
            n156 = In Range and Coerce(upper limit=1.0, x=w475, lower limit=-1.0) -> (In Range?=w479:bool)  [unwired: 1 out]
            n157 = Greater Or Equal?(x=w497, y=0.0) -> (x >= y?=w500:bool)
            n158 = call-poly <vilib>:"WPI_RobotDriveArcadeDrive.vi"("Y axis value"=w494, "X axis value"=w495, "RobotDriveDevRef"=w511) -> ("RobotDriveDevRef"=w493:T16)  [unwired: 6 in, 2 out]
            n159 = Greater Or Equal?(x=w505, y=-130.0) -> (x >= y?=w501:bool)
            n160 = Or(x=w500, y=TRUE) -> (x .or. y?=w481:bool)
            n161 = Not(x=w484) -> (.not. x?=w485:bool)
            n162 = Or(x=w479, y=TRUE) -> (x .or. y?=w482:bool)
            n163 = And(x=w481, y=w482) -> (x .and. y?=w480:bool)
            n164 = And(x=w501, y=w480) -> (x .and. y?=w483:bool)
            n165 = And(x=w483, y=w484) -> (x .and. y?=w487:bool)
            n166 = And(x=w483, y=w485) -> (x .and. y?=w486:bool)
            n167 = call-poly <vilib>:"WPI_SolenoidSet.vi"("Value"=w487, "SolenoidDevRef"=w489) -> ()  [unwired: 8 in, 2 out]
            n168 = call-poly <vilib>:"WPI_SolenoidSet.vi"("Value"=w486, "SolenoidDevRef"=w488) -> ()  [unwired: 8 in, 2 out]
          }
          frame "Test" {
            w522 = TRUE
            n169 = call <vilib>:"WPI_GyroGetAngle.vi"("GyroDevRef"=w512) -> ("Angle"=w513:dbl)  [unwired: 6 in, 4 out]
            n170 = call <vilib>:"WPI_AccelerometerGetAcceleration.vi"("AccelerometerDevRef"=w541) -> ("Accelerations"=w540:T24)  [unwired: 8 in, 2 out]
            n171 = call <vilib>:"WPI_EncoderGet.vi"("EncoderDevRef"=w546) -> ("Distance"=w543:dbl, "EncoderDevRef"=w530:T7)  [unwired: 5 in, 4 out]
            n172 = call <vilib>:"WPI_EncoderGet.vi"("EncoderDevRef"=w545) -> ("Distance"=w544:dbl, "EncoderDevRef"=w529:T7)  [unwired: 5 in, 4 out]
            n173 = Unbundle(w540) -> ("Z-Axis"=w535:dbl)  [unwired: 2 out]
            n174 = call "True Straight - Arcade T Test.vi"("Fwd/Rev Joy"=-0.5, "Bypass"=FALSE, "Left/Right Joy"=0.0, "Left Encoder"=w543, "Right Encoder"=w544) -> ("Fwd/Rev Out"=w533:dbl, "Left/Right Out"=w532:dbl)  [unwired: 8 in, 1 out]
            n175 = In Range and Coerce(upper limit=1.0, x=w513, lower limit=-1.0) -> (In Range?=w517:bool)  [unwired: 1 out]
            n176 = Greater Or Equal?(x=w535, y=0.0) -> (x >= y?=w538:bool)
            n177 = call-poly <vilib>:"WPI_RobotDriveArcadeDrive.vi"("Y axis value"=w532, "X axis value"=w533, "RobotDriveDevRef"=w549) -> ("RobotDriveDevRef"=w531:T16)  [unwired: 6 in, 2 out]
            n178 = Greater Or Equal?(x=w543, y=-130.0) -> (x >= y?=w539:bool)
            n179 = Or(x=w538, y=TRUE) -> (x .or. y?=w519:bool)
            n180 = Not(x=w522) -> (.not. x?=w523:bool)
            n181 = Or(x=w517, y=TRUE) -> (x .or. y?=w520:bool)
            n182 = And(x=w519, y=w520) -> (x .and. y?=w518:bool)
            n183 = And(x=w539, y=w518) -> (x .and. y?=w521:bool)
            n184 = And(x=w521, y=w522) -> (x .and. y?=w525:bool)
            n185 = And(x=w521, y=w523) -> (x .and. y?=w524:bool)
            n186 = call-poly <vilib>:"WPI_SolenoidSet.vi"("Value"=w525, "SolenoidDevRef"=w527) -> ()  [unwired: 8 in, 2 out]
            n187 = call-poly <vilib>:"WPI_SolenoidSet.vi"("Value"=w524, "SolenoidDevRef"=w526) -> ()  [unwired: 8 in, 2 out]
          }
        }
      }
    }
    frame #4 {
      n188 = while {
        tunnel: w558 -> [w572]
        tunnel: [w571] -> w557
        tunnel: [w561] -> w552
        tunnel: w556 -> [w565]
        tunnel: [w565] -> w555
        tunnel: w551 -> [w560]
        tunnel: [w559] -> w550
        stop <- w568 stop-if-true
        n189 = call <vilib>:"WPI_GyroGetAngle.vi"("GyroDevRef"=w560) -> ("Angle"=w561:dbl, "GyroDevRef"=w559:T4)  [unwired: 6 in, 3 out]
        n190 = call "Gyro Map"("Signals"=w561) -> ("Scaled Signals"=w564:dynamicdata)  [unwired: 9 in, 1 out]
        n191 = In Range and Coerce(upper limit=0.5, x=w561, lower limit=-0.5) -> (In Range?=w567:bool)  [unwired: 1 out]
        n192 = call "Convert from Dynamic Data"("Dynamic Data Type"=w564) -> ("Scalar"=w563:dbl)  [unwired: 3 in]
        n193 = Not(x=w565) -> (.not. x?=w566:bool)
        n194 = Or(x=w566, y=w567) -> (x .or. y?=w568:bool)
        n195 = call-poly <vilib>:"WPI_RobotDriveArcadeDrive.vi"("Y axis value"=w563, "X axis value"=0.0, "RobotDriveDevRef"=w572) -> ("RobotDriveDevRef"=w571:T16)  [unwired: 6 in, 2 out]
      }
    }
    frame #5 {
      n196 = call <vilib>:"WPI_EncoderReset.vi"("EncoderDevRef"=w576) -> ("EncoderDevRef"=w575:T7)  [unwired: 9 in, 1 out]
      n197 = call <vilib>:"WPI_GyroReset.vi"("GyroDevRef"=w578) -> ("GyroDevRef"=w577:T4)  [unwired: 9 in, 1 out]
      n198 = call <vilib>:"WPI_EncoderReset.vi"("EncoderDevRef"=w574) -> ("EncoderDevRef"=w573:T7)  [unwired: 9 in, 1 out]
    }
    frame #6 {
      n199 = Select(t=w591, s=w583, f="\"None\"") -> (s? t:f=w590:string)
      n200 = while {
        tunnel: w584 -> [w602]
        tunnel: w593 -> [w601]
        tunnel: w592 -> [w600]
        tunnel: w590 -> [w598]
        tunnel: [w597] -> w588
        tunnel: [w596] -> w587
        tunnel: [w595] -> w586
        tunnel: [w594] -> w585
        stop <- w599 stop-if-true
        n201 = case shown="\"None\", Default" w598 {
          tunnel: w602 -> [w605 w623 w639 w655 w671 w687 w703]
          tunnel: w601 -> [w604 w620 w636 w652 w668 w684 w700]
          tunnel: w600 -> [w603 w619 w635 w651 w667 w683 w699]
          tunnel: [TRUE w611 w627 w643 w659 w675 w691] -> w599
          tunnel: [0 1 2 3 4 5 6] -> w597
          tunnel: [w605 w610 w626 w642 w658 w674 w690] -> w596
          tunnel: [w604 w609 w625 w641 w657 w673 w689] -> w595
          tunnel: [w603 w608 w624 w640 w656 w672 w688] -> w594
          frame "None", Default {
          }
          frame "Position 1" {
            n202 = call <vilib>:"WPI_EncoderGet.vi"("EncoderDevRef"=w620) -> ("Distance"=w617:dbl, "EncoderDevRef"=w609:T7)  [unwired: 5 in, 4 out]
            n203 = call <vilib>:"WPI_EncoderGet.vi"("EncoderDevRef"=w619) -> ("Distance"=w618:dbl, "EncoderDevRef"=w608:T7)  [unwired: 5 in, 4 out]
            n204 = call "True Straight - Arcade T Test.vi"("Fwd/Rev Joy"=-0.75, "Bypass"=FALSE, "Left/Right Joy"=0.0, "Left Encoder"=w617, "Right Encoder"=w618) -> ("Fwd/Rev Out"=w614:dbl, "Left/Right Out"=w613:dbl)  [unwired: 8 in, 1 out]
            n205 = call-poly <vilib>:"WPI_RobotDriveArcadeDrive.vi"("Y axis value"=w613, "X axis value"=w614, "RobotDriveDevRef"=w623) -> ("RobotDriveDevRef"=w610:T16)  [unwired: 6 in, 2 out]
            n206 = Greater Or Equal?(x=w617, y=-39.0) -> (x >= y?=w611:bool)
          }
          frame "Position 2" {
            n207 = call <vilib>:"WPI_EncoderGet.vi"("EncoderDevRef"=w636) -> ("Distance"=w633:dbl, "EncoderDevRef"=w625:T7)  [unwired: 5 in, 4 out]
            n208 = call <vilib>:"WPI_EncoderGet.vi"("EncoderDevRef"=w635) -> ("Distance"=w634:dbl, "EncoderDevRef"=w624:T7)  [unwired: 5 in, 4 out]
            n209 = call "True Straight - Arcade T Test.vi"("Fwd/Rev Joy"=-0.75, "Bypass"=FALSE, "Left/Right Joy"=0.0, "Left Encoder"=w633, "Right Encoder"=w634) -> ("Fwd/Rev Out"=w630:dbl, "Left/Right Out"=w629:dbl)  [unwired: 8 in, 1 out]
            n210 = call-poly <vilib>:"WPI_RobotDriveArcadeDrive.vi"("Y axis value"=w629, "X axis value"=w630, "RobotDriveDevRef"=w639) -> ("RobotDriveDevRef"=w626:T16)  [unwired: 6 in, 2 out]
            n211 = Greater Or Equal?(x=w633, y=-117.5) -> (x >= y?=w627:bool)
          }
          frame "Position 3" {
            n212 = call <vilib>:"WPI_EncoderGet.vi"("EncoderDevRef"=w652) -> ("Distance"=w649:dbl, "EncoderDevRef"=w641:T7)  [unwired: 5 in, 4 out]
            n213 = call <vilib>:"WPI_EncoderGet.vi"("EncoderDevRef"=w651) -> ("Distance"=w650:dbl, "EncoderDevRef"=w640:T7)  [unwired: 5 in, 4 out]
            n214 = call "True Straight - Arcade T Test.vi"("Fwd/Rev Joy"=-0.75, "Bypass"=FALSE, "Left/Right Joy"=0.0, "Left Encoder"=w649, "Right Encoder"=w650) -> ("Fwd/Rev Out"=w646:dbl, "Left/Right Out"=w645:dbl)  [unwired: 8 in, 1 out]
            n215 = call-poly <vilib>:"WPI_RobotDriveArcadeDrive.vi"("Y axis value"=w645, "X axis value"=w646, "RobotDriveDevRef"=w655) -> ("RobotDriveDevRef"=w642:T16)  [unwired: 6 in, 2 out]
            n216 = Greater Or Equal?(x=w649, y=-39.0) -> (x >= y?=w643:bool)
          }
          frame "Position 4" {
            n217 = call <vilib>:"WPI_EncoderGet.vi"("EncoderDevRef"=w668) -> ("Distance"=w665:dbl, "EncoderDevRef"=w657:T7)  [unwired: 5 in, 4 out]
            n218 = call <vilib>:"WPI_EncoderGet.vi"("EncoderDevRef"=w667) -> ("Distance"=w666:dbl, "EncoderDevRef"=w656:T7)  [unwired: 5 in, 4 out]
            n219 = call "True Straight - Arcade T Test.vi"("Fwd/Rev Joy"=-0.75, "Bypass"=FALSE, "Left/Right Joy"=0.0, "Left Encoder"=w665, "Right Encoder"=w666) -> ("Fwd/Rev Out"=w662:dbl, "Left/Right Out"=w661:dbl)  [unwired: 8 in, 1 out]
            n220 = call-poly <vilib>:"WPI_RobotDriveArcadeDrive.vi"("Y axis value"=w661, "X axis value"=w662, "RobotDriveDevRef"=w671) -> ("RobotDriveDevRef"=w658:T16)  [unwired: 6 in, 2 out]
            n221 = Greater Or Equal?(x=w665, y=-58.0) -> (x >= y?=w659:bool)
          }
          frame "Position 5" {
            n222 = call <vilib>:"WPI_EncoderGet.vi"("EncoderDevRef"=w684) -> ("Distance"=w681:dbl, "EncoderDevRef"=w673:T7)  [unwired: 5 in, 4 out]
            n223 = call <vilib>:"WPI_EncoderGet.vi"("EncoderDevRef"=w683) -> ("Distance"=w682:dbl, "EncoderDevRef"=w672:T7)  [unwired: 5 in, 4 out]
            n224 = call "True Straight - Arcade T Test.vi"("Fwd/Rev Joy"=-0.75, "Bypass"=FALSE, "Left/Right Joy"=0.0, "Left Encoder"=w681, "Right Encoder"=w682) -> ("Fwd/Rev Out"=w678:dbl, "Left/Right Out"=w677:dbl)  [unwired: 8 in, 1 out]
            n225 = call-poly <vilib>:"WPI_RobotDriveArcadeDrive.vi"("Y axis value"=w677, "X axis value"=w678, "RobotDriveDevRef"=w687) -> ("RobotDriveDevRef"=w674:T16)  [unwired: 6 in, 2 out]
            n226 = Greater Or Equal?(x=w681, y=-39.0) -> (x >= y?=w675:bool)
          }
          frame "Test" {
            n227 = call <vilib>:"WPI_EncoderGet.vi"("EncoderDevRef"=w700) -> ("Distance"=w697:dbl, "EncoderDevRef"=w689:T7)  [unwired: 5 in, 4 out]
            n228 = call <vilib>:"WPI_EncoderGet.vi"("EncoderDevRef"=w699) -> ("Distance"=w698:dbl, "EncoderDevRef"=w688:T7)  [unwired: 5 in, 4 out]
            n229 = call "True Straight - Arcade T Test.vi"("Fwd/Rev Joy"=-0.75, "Bypass"=FALSE, "Left/Right Joy"=0.0, "Left Encoder"=w697, "Right Encoder"=w698) -> ("Fwd/Rev Out"=w694:dbl, "Left/Right Out"=w693:dbl)  [unwired: 8 in, 1 out]
            n230 = call-poly <vilib>:"WPI_RobotDriveArcadeDrive.vi"("Y axis value"=w693, "X axis value"=w694, "RobotDriveDevRef"=w703) -> ("RobotDriveDevRef"=w690:T16)  [unwired: 6 in, 2 out]
            n231 = Greater Or Equal?(x=w697, y=-161.0) -> (x >= y?=w691:bool)
          }
        }
      }
    }
    frame #7 {
      n232 = while {
        tunnel: w711 -> [w718]
        tunnel: w710 -> [w717]
        tunnel: [w715] -> w709
        tunnel: [w714] -> w708
        tunnel: w705 -> [w713]
        tunnel: [w712] -> w704
        stop <- w716 stop-if-true
        n233 = case shown="0, Default" w718 {
          selector: w718 -> [w722 w731 w739 w749 w757 w767 w781]
          tunnel: w717 -> [w720 w734 w740 w752 w758 w770 w784]
          tunnel: [TRUE w732 TRUE w750 TRUE w768 w782] -> w716
          tunnel: [w722 w731 w739 w749 w757 w767 w781] -> w715
          tunnel: [w720 w730 w740 w748 w758 w766 w780] -> w714
          tunnel: w713 -> [w719 w724 w738 w747 w755 w765 w779]
          tunnel: [w719 w723 w738 w741 w755 w759 w773] -> w712
          frame 0, Default {
          }
          frame 1 {
            w729 = 0.5
            w726 = 35.0
            n234 = call <vilib>:"WPI_GyroGetAngle.vi"("GyroDevRef"=w724) -> ("Angle"=w725:dbl, "GyroDevRef"=w723:T4)  [unwired: 6 in, 3 out]
            n235 = Subtract(x=w726, y=w725) -> (x-y=w733:dbl)
            n236 = call "Gyro Map2"("Signals"=w733) -> ("Scaled Signals"=w736:dynamicdata)  [unwired: 9 in, 1 out]
            n237 = call "Convert from Dynamic Data2"("Dynamic Data Type"=w736) -> ("Scalar"=w735:dbl)  [unwired: 3 in]
            n238 = Subtract(x=w726, y=w729) -> (x-y=w727:dbl)
            n239 = Add(x=w729, y=w726) -> (x+y=w728:dbl)
            n240 = call-poly <vilib>:"WPI_RobotDriveArcadeDrive.vi"("Y axis value"=w735, "RobotDriveDevRef"=w734) -> ("RobotDriveDevRef"=w730:T16)  [unwired: 7 in, 2 out]
            n241 = In Range and Coerce(upper limit=w728, x=w725, lower limit=w727) -> (In Range?=w732:bool)  [unwired: 1 out]
          }
          frame 2 {
          }
          frame 3 {
            w745 = 0.5
            w742 = -31.0
            n242 = call <vilib>:"WPI_GyroGetAngle.vi"("GyroDevRef"=w747) -> ("Angle"=w746:dbl, "GyroDevRef"=w741:T4)  [unwired: 6 in, 3 out]
            n243 = Subtract(x=w742, y=w746) -> (x-y=w751:dbl)
            n244 = call "Gyro Map4"("Signals"=w751) -> ("Scaled Signals"=w754:dynamicdata)  [unwired: 9 in, 1 out]
            n245 = Subtract(x=w742, y=w745) -> (x-y=w743:dbl)
            n246 = Add(x=w745, y=w742) -> (x+y=w744:dbl)
            n247 = call "Convert from Dynamic Data4"("Dynamic Data Type"=w754) -> ("Scalar"=w753:dbl)  [unwired: 3 in]
            n248 = In Range and Coerce(upper limit=w744, x=w746, lower limit=w743) -> (In Range?=w750:bool)  [unwired: 1 out]
            n249 = call-poly <vilib>:"WPI_RobotDriveArcadeDrive.vi"("Y axis value"=w753, "RobotDriveDevRef"=w752) -> ("RobotDriveDevRef"=w748:T16)  [unwired: 7 in, 2 out]
          }
          frame 4 {
          }
          frame 5 {
            w763 = 0.5
            w760 = -90.0
            n250 = call <vilib>:"WPI_GyroGetAngle.vi"("GyroDevRef"=w765) -> ("Angle"=w764:dbl, "GyroDevRef"=w759:T4)  [unwired: 6 in, 3 out]
            n251 = Subtract(x=w760, y=w764) -> (x-y=w769:dbl)
            n252 = call "Gyro Map6"("Signals"=w769) -> ("Scaled Signals"=w772:dynamicdata)  [unwired: 9 in, 1 out]
            n253 = Subtract(x=w760, y=w763) -> (x-y=w762:dbl)
            n254 = Add(x=w763, y=w760) -> (x+y=w761:dbl)
            n255 = call "Convert from Dynamic Data6"("Dynamic Data Type"=w772) -> ("Scalar"=w771:dbl)  [unwired: 3 in]
            n256 = In Range and Coerce(upper limit=w761, x=w764, lower limit=w762) -> (In Range?=w768:bool)  [unwired: 1 out]
            n257 = call-poly <vilib>:"WPI_RobotDriveArcadeDrive.vi"("Y axis value"=w771, "RobotDriveDevRef"=w770) -> ("RobotDriveDevRef"=w766:T16)  [unwired: 7 in, 2 out]
          }
          frame 6 {
            w777 = 0.5
            w774 = 34.0
            n258 = call <vilib>:"WPI_GyroGetAngle.vi"("GyroDevRef"=w779) -> ("Angle"=w778:dbl, "GyroDevRef"=w773:T4)  [unwired: 6 in, 3 out]
            n259 = Subtract(x=w774, y=w778) -> (x-y=w783:dbl)
            n260 = call "Gyro Map12"("Signals"=w783) -> ("Scaled Signals"=w786:dynamicdata)  [unwired: 9 in, 1 out]
            n261 = Subtract(x=w774, y=w777) -> (x-y=w776:dbl)
            n262 = Add(x=w777, y=w774) -> (x+y=w775:dbl)
            n263 = call "Convert from Dynamic Data12"("Dynamic Data Type"=w786) -> ("Scalar"=w785:dbl)  [unwired: 3 in]
            n264 = In Range and Coerce(upper limit=w775, x=w778, lower limit=w776) -> (In Range?=w782:bool)  [unwired: 1 out]
            n265 = call-poly <vilib>:"WPI_RobotDriveArcadeDrive.vi"("Y axis value"=w785, "RobotDriveDevRef"=w784) -> ("RobotDriveDevRef"=w780:T16)  [unwired: 7 in, 2 out]
          }
        }
      }
    }
    frame #8 {
      n266 = call <vilib>:"WPI_EncoderReset.vi"("EncoderDevRef"=w792) -> ("EncoderDevRef"=w791:T7)  [unwired: 9 in, 1 out]
      n267 = call <vilib>:"WPI_GyroReset.vi"("GyroDevRef"=w788) -> ("GyroDevRef"=w787:T4)  [unwired: 9 in, 1 out]
      n268 = call <vilib>:"WPI_EncoderReset.vi"("EncoderDevRef"=w790) -> ("EncoderDevRef"=w789:T7)  [unwired: 9 in, 1 out]
    }
    frame #9 {
      n269 = while {
        tunnel: w801 -> [w808]
        tunnel: w800 -> [w807]
        tunnel: w799 -> [w806]
        tunnel: w798 -> [w805]
        tunnel: [w803] -> w797
        tunnel: [w802] -> w796
        stop <- w804 stop-if-true
        n270 = case shown="0, Default" w808 {
          selector: w808 -> [w809 w812 w827 w829 w844 w846 w860]
          tunnel: w807 -> [w810 w817 w828 w834 w845 w851 w865]
          tunnel: w806 -> [_ w816 _ w833 _ w850 w864]
          tunnel: w805 -> [_ w815 _ w832 _ w849 w863]
          tunnel: [TRUE w814 TRUE w831 TRUE w848 w862] -> w804
          tunnel: [w810 w813 w828 w830 w845 w847 w861] -> w803
          tunnel: [w809 w812 w827 w829 w844 w846 w860] -> w802
          frame 0, Default {
          }
          frame 1 {
            n271 = call <vilib>:"WPI_EncoderGet.vi"("EncoderDevRef"=w816) -> ("Distance"=w822:dbl)  [unwired: 5 in, 5 out]
            n272 = call <vilib>:"WPI_EncoderGet.vi"("EncoderDevRef"=w815) -> ("Distance"=w823:dbl)  [unwired: 5 in, 5 out]
            n273 = call "True Straight - Arcade T Test.vi"("Fwd/Rev Joy"=-0.75, "Bypass"=FALSE, "Left/Right Joy"=0.0, "Left Encoder"=w822, "Right Encoder"=w823) -> ("Fwd/Rev Out"=w819:dbl, "Left/Right Out"=w818:dbl)  [unwired: 8 in, 1 out]
            n274 = call-poly <vilib>:"WPI_RobotDriveArcadeDrive.vi"("Y axis value"=w818, "X axis value"=w819, "RobotDriveDevRef"=w817) -> ("RobotDriveDevRef"=w813:T16)  [unwired: 6 in, 2 out]
            n275 = Greater Or Equal?(x=w822, y=-93.5) -> (x >= y?=w814:bool)
          }
          frame 2 {
          }
          frame 3 {
            n276 = call <vilib>:"WPI_EncoderGet.vi"("EncoderDevRef"=w833) -> ("Distance"=w839:dbl)  [unwired: 5 in, 5 out]
            n277 = call <vilib>:"WPI_EncoderGet.vi"("EncoderDevRef"=w832) -> ("Distance"=w840:dbl)  [unwired: 5 in, 5 out]
            n278 = call "True Straight - Arcade T Test.vi"("Fwd/Rev Joy"=-0.75, "Bypass"=FALSE, "Left/Right Joy"=0.0, "Left Encoder"=w839, "Right Encoder"=w840) -> ("Fwd/Rev Out"=w836:dbl, "Left/Right Out"=w835:dbl)  [unwired: 8 in, 1 out]
            n279 = call-poly <vilib>:"WPI_RobotDriveArcadeDrive.vi"("Y axis value"=w835, "X axis value"=w836, "RobotDriveDevRef"=w834) -> ("RobotDriveDevRef"=w830:T16)  [unwired: 6 in, 2 out]
            n280 = Greater Or Equal?(x=w839, y=-94.0) -> (x >= y?=w831:bool)
          }
          frame 4 {
          }
          frame 5 {
            n281 = call <vilib>:"WPI_EncoderGet.vi"("EncoderDevRef"=w850) -> ("Distance"=w856:dbl)  [unwired: 5 in, 5 out]
            n282 = call <vilib>:"WPI_EncoderGet.vi"("EncoderDevRef"=w849) -> ("Distance"=w857:dbl)  [unwired: 5 in, 5 out]
            n283 = call "True Straight - Arcade T Test.vi"("Fwd/Rev Joy"=-0.75, "Bypass"=FALSE, "Left/Right Joy"=0.0, "Left Encoder"=w856, "Right Encoder"=w857) -> ("Fwd/Rev Out"=w853:dbl, "Left/Right Out"=w852:dbl)  [unwired: 8 in, 1 out]
            n284 = call-poly <vilib>:"WPI_RobotDriveArcadeDrive.vi"("Y axis value"=w852, "X axis value"=w853, "RobotDriveDevRef"=w851) -> ("RobotDriveDevRef"=w847:T16)  [unwired: 6 in, 2 out]
            n285 = Greater Or Equal?(x=w856, y=-64.5) -> (x >= y?=w848:bool)
          }
          frame 6 {
            n286 = call <vilib>:"WPI_EncoderGet.vi"("EncoderDevRef"=w864) -> ("Distance"=w870:dbl)  [unwired: 5 in, 5 out]
            n287 = call <vilib>:"WPI_EncoderGet.vi"("EncoderDevRef"=w863) -> ("Distance"=w871:dbl)  [unwired: 5 in, 5 out]
            n288 = call "True Straight - Arcade T Test.vi"("Fwd/Rev Joy"=-0.75, "Bypass"=FALSE, "Left/Right Joy"=0.0, "Left Encoder"=w870, "Right Encoder"=w871) -> ("Fwd/Rev Out"=w867:dbl, "Left/Right Out"=w866:dbl)  [unwired: 8 in, 1 out]
            n289 = call-poly <vilib>:"WPI_RobotDriveArcadeDrive.vi"("Y axis value"=w866, "X axis value"=w867, "RobotDriveDevRef"=w865) -> ("RobotDriveDevRef"=w861:T16)  [unwired: 6 in, 2 out]
            n290 = Greater Or Equal?(x=w870, y=-177.0) -> (x >= y?=w862:bool)
          }
        }
      }
    }
    frame #10 {
      n291 = while {
        tunnel: w876 -> [w883]
        tunnel: w877 -> [w882]
        tunnel: [w880] -> _
        tunnel: [w879] -> w874
        tunnel: w875 -> [w878]
        stop <- w881 stop-if-true
        n292 = case shown="0, Default" w883 {
          selector: w883 -> [w886 w894 w907 w920 w933 w946 w959]
          tunnel: w882 -> [w884 w897 w910 w923 w936 w949 w962]
          tunnel: [TRUE w895 w908 w921 w934 w947 w960] -> w881
          tunnel: [w886 w894 w907 w920 w933 w946 w959] -> w880
          tunnel: [w884 w893 w906 w919 w932 w945 w958] -> w879
          tunnel: w878 -> [_ w887 w902 w918 w931 w944 w957]
          frame 0, Default {
          }
          frame 1 {
            w892 = 0.5
            w889 = -156.0
            n293 = call <vilib>:"WPI_GyroGetAngle.vi"("GyroDevRef"=w887) -> ("Angle"=w888:dbl)  [unwired: 6 in, 4 out]
            n294 = Subtract(x=w889, y=w888) -> (x-y=w896:dbl)
            n295 = call "Gyro Map7"("Signals"=w896) -> ("Scaled Signals"=w899:dynamicdata)  [unwired: 9 in, 1 out]
            n296 = call "Convert from Dynamic Data7"("Dynamic Data Type"=w899) -> ("Scalar"=w898:dbl)  [unwired: 3 in]
            n297 = Subtract(x=w889, y=w892) -> (x-y=w890:dbl)
            n298 = Add(x=w892, y=w889) -> (x+y=w891:dbl)
            n299 = call-poly <vilib>:"WPI_RobotDriveArcadeDrive.vi"("Y axis value"=w898, "RobotDriveDevRef"=w897) -> ("RobotDriveDevRef"=w893:T16)  [unwired: 7 in, 2 out]
            n300 = In Range and Coerce(upper limit=w891, x=w888, lower limit=w890) -> (In Range?=w895:bool)  [unwired: 1 out]
          }
          frame 2 {
            w901 = -120.0
            w905 = 0.5
            n301 = call <vilib>:"WPI_GyroGetAngle.vi"("GyroDevRef"=w902) -> ("Angle"=w900:dbl)  [unwired: 6 in, 4 out]
            n302 = Subtract(x=w901, y=w900) -> (x-y=w909:dbl)
            n303 = call "Gyro Map8"("Signals"=w909) -> ("Scaled Signals"=w912:dynamicdata)  [unwired: 9 in, 1 out]
            n304 = Subtract(x=w901, y=w905) -> (x-y=w904:dbl)
            n305 = Add(x=w905, y=w901) -> (x+y=w903:dbl)
            n306 = call "Convert from Dynamic Data8"("Dynamic Data Type"=w912) -> ("Scalar"=w911:dbl)  [unwired: 3 in]
            n307 = In Range and Coerce(upper limit=w903, x=w900, lower limit=w904) -> (In Range?=w908:bool)  [unwired: 1 out]
            n308 = call-poly <vilib>:"WPI_RobotDriveArcadeDrive.vi"("Y axis value"=w911, "RobotDriveDevRef"=w910) -> ("RobotDriveDevRef"=w906:T16)  [unwired: 7 in, 2 out]
          }
          frame 3 {
            w916 = 0.5
            w913 = -89.0
            n309 = call <vilib>:"WPI_GyroGetAngle.vi"("GyroDevRef"=w918) -> ("Angle"=w917:dbl)  [unwired: 6 in, 4 out]
            n310 = Subtract(x=w913, y=w917) -> (x-y=w922:dbl)
            n311 = call "Gyro Map9"("Signals"=w922) -> ("Scaled Signals"=w925:dynamicdata)  [unwired: 9 in, 1 out]
            n312 = Subtract(x=w913, y=w916) -> (x-y=w914:dbl)
            n313 = Add(x=w916, y=w913) -> (x+y=w915:dbl)
            n314 = call "Convert from Dynamic Data9"("Dynamic Data Type"=w925) -> ("Scalar"=w924:dbl)  [unwired: 3 in]
            n315 = In Range and Coerce(upper limit=w915, x=w917, lower limit=w914) -> (In Range?=w921:bool)  [unwired: 1 out]
            n316 = call-poly <vilib>:"WPI_RobotDriveArcadeDrive.vi"("Y axis value"=w924, "RobotDriveDevRef"=w923) -> ("RobotDriveDevRef"=w919:T16)  [unwired: 7 in, 2 out]
          }
          frame 4 {
            w929 = 0.5
            w926 = 175.0
            n317 = call <vilib>:"WPI_GyroGetAngle.vi"("GyroDevRef"=w931) -> ("Angle"=w930:dbl)  [unwired: 6 in, 4 out]
            n318 = Subtract(x=w926, y=w930) -> (x-y=w935:dbl)
            n319 = call "Gyro Map10"("Signals"=w935) -> ("Scaled Signals"=w938:dynamicdata)  [unwired: 9 in, 1 out]
            n320 = Subtract(x=w926, y=w929) -> (x-y=w927:dbl)
            n321 = Add(x=w929, y=w926) -> (x+y=w928:dbl)
            n322 = call "Convert from Dynamic Data10"("Dynamic Data Type"=w938) -> ("Scalar"=w937:dbl)  [unwired: 3 in]
            n323 = In Range and Coerce(upper limit=w928, x=w930, lower limit=w927) -> (In Range?=w934:bool)  [unwired: 1 out]
            n324 = call-poly <vilib>:"WPI_RobotDriveArcadeDrive.vi"("Y axis value"=w937, "RobotDriveDevRef"=w936) -> ("RobotDriveDevRef"=w932:T16)  [unwired: 7 in, 2 out]
          }
          frame 5 {
            w942 = 0.5
            w939 = -90.0
            n325 = call <vilib>:"WPI_GyroGetAngle.vi"("GyroDevRef"=w944) -> ("Angle"=w943:dbl)  [unwired: 6 in, 4 out]
            n326 = Subtract(x=w939, y=w943) -> (x-y=w948:dbl)
            n327 = call "Gyro Map11"("Signals"=w948) -> ("Scaled Signals"=w951:dynamicdata)  [unwired: 9 in, 1 out]
            n328 = Subtract(x=w939, y=w942) -> (x-y=w941:dbl)
            n329 = Add(x=w942, y=w939) -> (x+y=w940:dbl)
            n330 = call "Convert from Dynamic Data11"("Dynamic Data Type"=w951) -> ("Scalar"=w950:dbl)  [unwired: 3 in]
            n331 = In Range and Coerce(upper limit=w940, x=w943, lower limit=w941) -> (In Range?=w947:bool)  [unwired: 1 out]
            n332 = call-poly <vilib>:"WPI_RobotDriveArcadeDrive.vi"("Y axis value"=w950, "RobotDriveDevRef"=w949) -> ("RobotDriveDevRef"=w945:T16)  [unwired: 7 in, 2 out]
          }
          frame 6 {
            w955 = 0.5
            w952 = 34.0
            n333 = call <vilib>:"WPI_GyroGetAngle.vi"("GyroDevRef"=w957) -> ("Angle"=w956:dbl)  [unwired: 6 in, 4 out]
            n334 = Subtract(x=w952, y=w956) -> (x-y=w961:dbl)
            n335 = call "Gyro Map13"("Signals"=w961) -> ("Scaled Signals"=w964:dynamicdata)  [unwired: 9 in, 1 out]
            n336 = Subtract(x=w952, y=w955) -> (x-y=w954:dbl)
            n337 = Add(x=w955, y=w952) -> (x+y=w953:dbl)
            n338 = call "Convert from Dynamic Data13"("Dynamic Data Type"=w964) -> ("Scalar"=w963:dbl)  [unwired: 3 in]
            n339 = In Range and Coerce(upper limit=w953, x=w956, lower limit=w954) -> (In Range?=w960:bool)  [unwired: 1 out]
            n340 = call-poly <vilib>:"WPI_RobotDriveArcadeDrive.vi"("Y axis value"=w963, "RobotDriveDevRef"=w962) -> ("RobotDriveDevRef"=w958:T16)  [unwired: 7 in, 2 out]
          }
        }
      }
    }
    frame #11 {
      n341 = while {
        tunnel: w971 -> [w979]
        tunnel: w970 -> [w978]
        tunnel: w969 -> [w976]
        tunnel: w968 -> [w975]
        tunnel: w967 -> [w974]
        tunnel: w966 -> [w973]
        tunnel: w965 -> [w972]
        stop <- w977 stop-if-true
        n342 = case shown="\"Low Bar\"" w979 {
          tunnel: w978 -> [_ w1007 _ _ w1166 w1321 _ _ w1478 w1633 w1788]
          tunnel: [TRUE w982 TRUE TRUE w1138 w1293 TRUE TRUE w1450 w1605 w1763] -> w977
          tunnel: w976 -> [_ w1006 _ _ w1142 w1302 _ _ w1456 w1612 w1767]
          tunnel: w975 -> [_ w983 _ _ w1140 w1295 _ _ w1452 w1607 w1760]
          tunnel: w974 -> [_ w998 _ _ w1145 w1301 _ _ w1457 w1611 w1766]
          tunnel: w973 -> [_ w991 _ _ w1146 w1299 _ _ w1458 w1613 w1769]
          tunnel: w972 -> [_ w990 _ _ w1147 w1300 _ _ w1459 w1614 w1768]
          frame "None", Default {
          }
          frame "Low Bar" {
            n343 = global read "Global 2.vi" "Cam Y Pos"() -> (w1000:dbl)
            n344 = global read "Global 1.vi" "Cam X Pos"() -> (w999:dbl)
            n345 = call <vilib>:"WPI_ServoSetPosition.vi"("Position"=180, "ServoDeviceRef"=w1006) -> ()  [unwired: 8 in, 2 out]
            n346 = call "Camera Positioning 2.vi"("Aim"=w983, "Y Position"=w1000, "X Position"=w999) -> ("Aim Finished"=w988:bool, "Fwd/Rev Out"=w996:dbl, "Left/Right Out"=w997:dbl)  [unwired: 6 in]
            n347 = Select(t=enum16{"Off", "On", "Forward", "Reverse"}."Forward", s=w983, f=enum16{"Off", "On", "Forward", "Reverse"}."Off") -> (s? t:f=w1002:enum16{"Off", "On", "Forward", "Reverse"})
            n348 = call-poly <vilib>:"WPI_RobotDriveArcadeDrive.vi"("Y axis value"=w997, "X axis value"=w996, "RobotDriveDevRef"=w1007) -> ()  [unwired: 6 in, 3 out]
            n349 = call <vilib>:"WPI_RelaySet.vi"("RelayValue"=w1002, "RelayDevRef"=w998) -> ()  [unwired: 8 in, 2 out]
            n350 = xnode "Timer On Delay"("preset time (ms)"=1000, "input"=w988) -> ("output"=w985:bool)  [unwired: 1 in, 2 out]
            n351 = call-poly <vilib>:"NT Write Value.vi"("Boolean"=w988, "Name"="Aimed!") -> ()  [unwired: 9 in, 1 out]
            n352 = xnode "Pulse Timer"("preset time (ms)"=1000, "input"=w985) -> ("output"=w981:bool)  [unwired: 1 in, 2 out]
            n353 = Not(x=w983) -> (.not. x?=w984:bool)
            n354 = xnode "Pulse Timer"("preset time (ms)"=500, "input"=w983) -> ("output"=w989:bool)  [unwired: 1 in, 2 out]
            n355 = And(x=w989, y=TRUE) -> (x .and. y?=w1009:bool)
            n356 = Select(t=-1.0, s=w981, f=0.0) -> (s? t:f=w994:dbl)
            n357 = call-poly <vilib>:"WPI_SolenoidSet.vi"("Value"=w1009, "SolenoidDevRef"=w991) -> ()  [unwired: 8 in, 2 out]
            n358 = call <vilib>:"WPI_MotorControlSetOutput.vi"("Output"=w994, "MotorControlDevRef"=w990) -> ()  [unwired: 7 in, 3 out]
            n359 = Or(x=w981, y=w984) -> (x .or. y?=w982:bool)
          }
          frame "Portcullis" {
          }
          frame "Cheval" {
          }
          frame "Ramparts" {
            n360 = global read "Global 2.vi" "Cam Y Pos"() -> (w1158:dbl)
            n361 = global read "Global 1.vi" "Cam X Pos"() -> (w1157:dbl)
            n362 = call <vilib>:"WPI_ServoSetPosition.vi"("Position"=180, "ServoDeviceRef"=w1142) -> ()  [unwired: 8 in, 2 out]
            n363 = call "Camera Positioning 2.vi"("Aim"=w1140, "Y Position"=w1158, "X Position"=w1157) -> ("Aim Finished"=w1151:bool, "Fwd/Rev Out"=w1143:dbl, "Left/Right Out"=w1144:dbl)  [unwired: 6 in]
            n364 = Select(t=enum16{"Off", "On", "Forward", "Reverse"}."Forward", s=w1140, f=enum16{"Off", "On", "Forward", "Reverse"}."Off") -> (s? t:f=w1160:enum16{"Off", "On", "Forward", "Reverse"})
            n365 = call-poly <vilib>:"WPI_RobotDriveArcadeDrive.vi"("Y axis value"=w1144, "X axis value"=w1143, "RobotDriveDevRef"=w1166) -> ()  [unwired: 6 in, 3 out]
            n366 = call <vilib>:"WPI_RelaySet.vi"("RelayValue"=w1160, "RelayDevRef"=w1145) -> ()  [unwired: 8 in, 2 out]
            n367 = xnode "Timer On Delay"("preset time (ms)"=1000, "input"=w1151) -> ("output"=w1148:bool)  [unwired: 1 in, 2 out]
            n368 = call-poly <vilib>:"NT Write Value.vi"("Boolean"=w1151, "Name"="Aimed!") -> ()  [unwired: 9 in, 1 out]
            n369 = Not(x=w1140) -> (.not. x?=w1141:bool)
            n370 = xnode "Pulse Timer"("preset time (ms)"=1000, "input"=w1148) -> ("output"=w1139:bool)  [unwired: 1 in, 2 out]
            n371 = xnode "Pulse Timer"("preset time (ms)"=500, "input"=w1140) -> ("output"=w1152:bool)  [unwired: 1 in, 2 out]
            n372 = And(x=w1152, y=TRUE) -> (x .and. y?=w1165:bool)
            n373 = Select(t=-1.0, s=w1139, f=0.0) -> (s? t:f=w1155:dbl)
            n374 = call-poly <vilib>:"WPI_SolenoidSet.vi"("Value"=w1165, "SolenoidDevRef"=w1146) -> ()  [unwired: 8 in, 2 out]
            n375 = call <vilib>:"WPI_MotorControlSetOutput.vi"("Output"=w1155, "MotorControlDevRef"=w1147) -> ()  [unwired: 7 in, 3 out]
            n376 = Or(x=w1139, y=w1141) -> (x .or. y?=w1138:bool)
          }
          frame "Moat" {
            n377 = global read "Global 2.vi" "Cam Y Pos"() -> (w1313:dbl)
            n378 = global read "Global 1.vi" "Cam X Pos"() -> (w1312:dbl)
            n379 = call <vilib>:"WPI_ServoSetPosition.vi"("Position"=180, "ServoDeviceRef"=w1302) -> ()  [unwired: 8 in, 2 out]
            n380 = call "Camera Positioning 2.vi"("Aim"=w1295, "Y Position"=w1313, "X Position"=w1312) -> ("Aim Finished"=w1306:bool, "Fwd/Rev Out"=w1297:dbl, "Left/Right Out"=w1298:dbl)  [unwired: 6 in]
            n381 = Select(t=enum16{"Off", "On", "Forward", "Reverse"}."Forward", s=w1295, f=enum16{"Off", "On", "Forward", "Reverse"}."Off") -> (s? t:f=w1315:enum16{"Off", "On", "Forward", "Reverse"})
            n382 = call-poly <vilib>:"WPI_RobotDriveArcadeDrive.vi"("Y axis value"=w1298, "X axis value"=w1297, "RobotDriveDevRef"=w1321) -> ()  [unwired: 6 in, 3 out]
            n383 = call <vilib>:"WPI_RelaySet.vi"("RelayValue"=w1315, "RelayDevRef"=w1301) -> ()  [unwired: 8 in, 2 out]
            n384 = xnode "Timer On Delay"("preset time (ms)"=1000, "input"=w1306) -> ("output"=w1303:bool)  [unwired: 1 in, 2 out]
            n385 = call-poly <vilib>:"NT Write Value.vi"("Boolean"=w1306, "Name"="Aimed!") -> ()  [unwired: 9 in, 1 out]
            n386 = Not(x=w1295) -> (.not. x?=w1296:bool)
            n387 = xnode "Pulse Timer"("preset time (ms)"=1000, "input"=w1303) -> ("output"=w1294:bool)  [unwired: 1 in, 2 out]
            n388 = xnode "Pulse Timer"("preset time (ms)"=500, "input"=w1295) -> ("output"=w1307:bool)  [unwired: 1 in, 2 out]
            n389 = And(x=w1307, y=TRUE) -> (x .and. y?=w1320:bool)
            n390 = Select(t=-1.0, s=w1294, f=0.0) -> (s? t:f=w1310:dbl)
            n391 = call-poly <vilib>:"WPI_SolenoidSet.vi"("Value"=w1320, "SolenoidDevRef"=w1299) -> ()  [unwired: 8 in, 2 out]
            n392 = call <vilib>:"WPI_MotorControlSetOutput.vi"("Output"=w1310, "MotorControlDevRef"=w1300) -> ()  [unwired: 7 in, 3 out]
            n393 = Or(x=w1294, y=w1296) -> (x .or. y?=w1293:bool)
          }
          frame "Drawbridge" {
          }
          frame "Sally Port" {
          }
          frame "Rock Wall" {
            n394 = global read "Global 2.vi" "Cam Y Pos"() -> (w1470:dbl)
            n395 = global read "Global 1.vi" "Cam X Pos"() -> (w1469:dbl)
            n396 = call <vilib>:"WPI_ServoSetPosition.vi"("Position"=180, "ServoDeviceRef"=w1456) -> ()  [unwired: 8 in, 2 out]
            n397 = call "Camera Positioning 2.vi"("Aim"=w1452, "Y Position"=w1470, "X Position"=w1469) -> ("Aim Finished"=w1463:bool, "Fwd/Rev Out"=w1455:dbl, "Left/Right Out"=w1454:dbl)  [unwired: 6 in]
            n398 = Select(t=enum16{"Off", "On", "Forward", "Reverse"}."Forward", s=w1452, f=enum16{"Off", "On", "Forward", "Reverse"}."Off") -> (s? t:f=w1472:enum16{"Off", "On", "Forward", "Reverse"})
            n399 = call-poly <vilib>:"WPI_RobotDriveArcadeDrive.vi"("Y axis value"=w1454, "X axis value"=w1455, "RobotDriveDevRef"=w1478) -> ()  [unwired: 6 in, 3 out]
            n400 = call <vilib>:"WPI_RelaySet.vi"("RelayValue"=w1472, "RelayDevRef"=w1457) -> ()  [unwired: 8 in, 2 out]
            n401 = xnode "Timer On Delay"("preset time (ms)"=1000, "input"=w1463) -> ("output"=w1460:bool)  [unwired: 1 in, 2 out]
            n402 = call-poly <vilib>:"NT Write Value.vi"("Boolean"=w1463, "Name"="Aimed!") -> ()  [unwired: 9 in, 1 out]
            n403 = Not(x=w1452) -> (.not. x?=w1453:bool)
            n404 = xnode "Pulse Timer"("preset time (ms)"=1000, "input"=w1460) -> ("output"=w1451:bool)  [unwired: 1 in, 2 out]
            n405 = xnode "Pulse Timer"("preset time (ms)"=500, "input"=w1452) -> ("output"=w1464:bool)  [unwired: 1 in, 2 out]
            n406 = And(x=w1464, y=TRUE) -> (x .and. y?=w1477:bool)
            n407 = Select(t=-1.0, s=w1451, f=0.0) -> (s? t:f=w1467:dbl)
            n408 = call-poly <vilib>:"WPI_SolenoidSet.vi"("Value"=w1477, "SolenoidDevRef"=w1458) -> ()  [unwired: 8 in, 2 out]
            n409 = call <vilib>:"WPI_MotorControlSetOutput.vi"("Output"=w1467, "MotorControlDevRef"=w1459) -> ()  [unwired: 7 in, 3 out]
            n410 = Or(x=w1451, y=w1453) -> (x .or. y?=w1450:bool)
          }
          frame "Rough Terrain" {
            n411 = global read "Global 2.vi" "Cam Y Pos"() -> (w1625:dbl)
            n412 = global read "Global 1.vi" "Cam X Pos"() -> (w1624:dbl)
            n413 = call <vilib>:"WPI_ServoSetPosition.vi"("Position"=180, "ServoDeviceRef"=w1612) -> ()  [unwired: 8 in, 2 out]
            n414 = call "Camera Positioning 2.vi"("Aim"=w1607, "Y Position"=w1625, "X Position"=w1624) -> ("Aim Finished"=w1618:bool, "Fwd/Rev Out"=w1610:dbl, "Left/Right Out"=w1609:dbl)  [unwired: 6 in]
            n415 = Select(t=enum16{"Off", "On", "Forward", "Reverse"}."Forward", s=w1607, f=enum16{"Off", "On", "Forward", "Reverse"}."Off") -> (s? t:f=w1627:enum16{"Off", "On", "Forward", "Reverse"})
            n416 = call-poly <vilib>:"WPI_RobotDriveArcadeDrive.vi"("Y axis value"=w1609, "X axis value"=w1610, "RobotDriveDevRef"=w1633) -> ()  [unwired: 6 in, 3 out]
            n417 = call <vilib>:"WPI_RelaySet.vi"("RelayValue"=w1627, "RelayDevRef"=w1611) -> ()  [unwired: 8 in, 2 out]
            n418 = xnode "Timer On Delay"("preset time (ms)"=1000, "input"=w1618) -> ("output"=w1615:bool)  [unwired: 1 in, 2 out]
            n419 = call-poly <vilib>:"NT Write Value.vi"("Boolean"=w1618, "Name"="Aimed!") -> ()  [unwired: 9 in, 1 out]
            n420 = xnode "Pulse Timer"("preset time (ms)"=1000, "input"=w1615) -> ("output"=w1606:bool)  [unwired: 1 in, 2 out]
            n421 = Not(x=w1607) -> (.not. x?=w1608:bool)
            n422 = xnode "Pulse Timer"("preset time (ms)"=500, "input"=w1607) -> ("output"=w1619:bool)  [unwired: 1 in, 2 out]
            n423 = And(x=w1619, y=TRUE) -> (x .and. y?=w1632:bool)
            n424 = Select(t=-1.0, s=w1606, f=0.0) -> (s? t:f=w1622:dbl)
            n425 = call-poly <vilib>:"WPI_SolenoidSet.vi"("Value"=w1632, "SolenoidDevRef"=w1613) -> ()  [unwired: 8 in, 2 out]
            n426 = call <vilib>:"WPI_MotorControlSetOutput.vi"("Output"=w1622, "MotorControlDevRef"=w1614) -> ()  [unwired: 7 in, 3 out]
            n427 = Or(x=w1606, y=w1608) -> (x .or. y?=w1605:bool)
          }
          frame "Test" {
            n428 = global read "Global 2.vi" "Cam Y Pos"() -> (w1780:dbl)
            n429 = global read "Global 1.vi" "Cam X Pos"() -> (w1779:dbl)
            n430 = call <vilib>:"WPI_ServoSetPosition.vi"("Position"=180, "ServoDeviceRef"=w1767) -> ()  [unwired: 8 in, 2 out]
            n431 = call "Camera Positioning 2.vi"("Aim"=w1760, "Y Position"=w1780, "X Position"=w1779) -> ("Aim Finished"=w1773:bool, "Fwd/Rev Out"=w1764:dbl, "Left/Right Out"=w1765:dbl)  [unwired: 6 in]
            n432 = Select(t=enum16{"Off", "On", "Forward", "Reverse"}."Forward", s=w1760, f=enum16{"Off", "On", "Forward", "Reverse"}."Off") -> (s? t:f=w1782:enum16{"Off", "On", "Forward", "Reverse"})
            n433 = call-poly <vilib>:"WPI_RobotDriveArcadeDrive.vi"("Y axis value"=w1765, "X axis value"=w1764, "RobotDriveDevRef"=w1788) -> ()  [unwired: 6 in, 3 out]
            n434 = call <vilib>:"WPI_RelaySet.vi"("RelayValue"=w1782, "RelayDevRef"=w1766) -> ()  [unwired: 8 in, 2 out]
            n435 = xnode "Timer On Delay"("preset time (ms)"=1000, "input"=w1773) -> ("output"=w1770:bool)  [unwired: 1 in, 2 out]
            n436 = call-poly <vilib>:"NT Write Value.vi"("Boolean"=w1773, "Name"="Aimed!") -> ()  [unwired: 9 in, 1 out]
            n437 = xnode "Pulse Timer"("preset time (ms)"=1000, "input"=w1770) -> ("output"=w1761:bool)  [unwired: 1 in, 2 out]
            n438 = Not(x=w1760) -> (.not. x?=w1762:bool)
            n439 = xnode "Pulse Timer"("preset time (ms)"=500, "input"=w1760) -> ("output"=w1774:bool)  [unwired: 1 in, 2 out]
            n440 = And(x=w1774, y=TRUE) -> (x .and. y?=w1787:bool)
            n441 = Select(t=-1.0, s=w1761, f=0.0) -> (s? t:f=w1777:dbl)
            n442 = call-poly <vilib>:"WPI_SolenoidSet.vi"("Value"=w1787, "SolenoidDevRef"=w1769) -> ()  [unwired: 8 in, 2 out]
            n443 = call <vilib>:"WPI_MotorControlSetOutput.vi"("Output"=w1777, "MotorControlDevRef"=w1768) -> ()  [unwired: 7 in, 3 out]
            n444 = Or(x=w1761, y=w1762) -> (x .or. y?=w1763:bool)
          }
        }
      }
    }
  }
  n445 = call <vilib>:"WPI_PotentiometerGetNormalized.vi"("error in"=w45, "PotDevRef"=w44) -> ("Normalized Value"=w2:dbl)  [unwired: 7 in, 2 out]
  n446 = call <vilib>:"WPI_JoystickGetValues.vi"("JoystickDevRef"=w100) -> ("Axes"=w98:dbl[])  [unwired: 6 in, 4 out]
  n447 = call-poly <vilib>:"NT Write Value.vi"("Numeric Array"=w98, "Name"="Joystick 0/Axes") -> ()  [unwired: 9 in, 1 out]
  n448 = Index Array(array=w98, index=2) -> ()  [unwired: 1 out]
  n449 = Multiply(x=w2, y=270.0) -> (x*y=w1:dbl)
  "Actual Arm Angle" <- w1
  n450 = call <vilib>:"WPI_SolenoidRefNum Registry Get.vi"("refnum name"="Extend Rear Wheels") -> ("SolenoidDevRef"=w61:T14)  [unwired: 9 in, 1 out]
  n451 = call <vilib>:"WPI_SolenoidRefNum Registry Get.vi"("refnum name"="Retract Rear Wheels") -> ("SolenoidDevRef"=w60:T14)  [unwired: 9 in, 1 out]
  n452 = call <vilib>:"WPI_SolenoidRefNum Registry Get.vi"("refnum name"="Low Speed") -> ("SolenoidDevRef"=w63:T14)  [unwired: 9 in, 1 out]
  n453 = disable-structure shown="Disabled" {
    frame Disabled {
      # "Use time and/or sensors to control how the robot drives."
      n454 = case shown="\"Alternative 1\"" {
        selector: _ -> [_ _ _ _ _ _ _ _ _ _ _ _ _ _]
        frame Default {
          # "You can put your main auto here, or you can right-click on the case and make any\nother frame be the default case."
          # "This is the frame that will execute if no selection is made, or if it is not recognized"
        }
        frame "Alternative 1" {
          # "This sample code describes robot movements in an array. You can extend it to control other motors\non your robot. You can also use file I/O to move the data to a text file."
          n455 = call <vilib>:"WPI_RobotDriveRefNum Registry Get.vi"("refnum name"="Left and Right Motors") -> ("RobotDriveDevRef"=w1916:T16)  [unwired: 1 in, 9 out]
          n456 = for {
            shift-right: [w1924] -> _
            shift-left: w1916 -> [w1925]
            tunnel: "Array of robot movements" -> [w1920] mode=indexing
            n457 = Unbundle By Name(w1920) -> ("X Joystick Value"=w1923:dbl, "Y Joystick Value"=w1922:dbl, "Delay (sec)"=w1921:dbl)  [unwired: 1 out]
            n458 = call-poly <vilib>:"WPI_RobotDriveArcadeDrive.vi"("Y axis value"=w1922, "X axis value"=w1923, "RobotDriveDevRef"=w1925) -> ("Motor Values"=w1918:dbl[], "RobotDriveDevRef"=w1926:T16)  [unwired: 1 in, 6 out]
            n459 = call-poly <vilib>:"NT Write Value.vi"("Numeric Array"=w1918, "Name"="RobotDrive Motors") -> ()  [unwired: 9 in, 1 out]
            n460 = call <vilib>:"WPI_RobotDriveDelayAndUpdateSafety.vi"("Delay (s)"=w1921, "RobotDriveDevRef"=w1926) -> ("RobotDriveDevRef 2"=w1924:T16)  [unwired: 8 in, 1 out]
            "Current Movement, for debugging" <- w1920
          }
        }
        frame "Alternative 2" {
          w1928 = "RobotDrive Motors" ("Name")
          # "This is some simple sample code to drive your robot curving one direction and then the other."
          # "stand still"
          # "other way for 0.5 second"
          # "turn for 1 second"
          n461 = call <vilib>:"WPI_RobotDriveRefNum Registry Get.vi"("refnum name"="Left and Right Motors") -> ("RobotDriveDevRef"=w1944:T16)  [unwired: 1 in, 9 out]
          n462 = call-poly <vilib>:"WPI_RobotDriveArcadeDrive.vi"("Y axis value"=0.5 ("X axis value"), "X axis value"=-0.25, "RobotDriveDevRef"=w1944) -> ("Motor Values"=w1927:dbl[], "RobotDriveDevRef"=w1937:T16)  [unwired: 1 in, 6 out]
          n463 = call-poly <vilib>:"NT Write Value.vi"("Numeric Array"=w1927, "Name"=w1928) -> ()  [unwired: 9 in, 1 out]
          n464 = call <vilib>:"WPI_RobotDriveDelayAndUpdateSafety.vi"("Delay (s)"=1.0, "RobotDriveDevRef"=w1937) -> ("RobotDriveDevRef 2"=w1938:T16)  [unwired: 8 in, 1 out]
          n465 = call-poly <vilib>:"WPI_RobotDriveArcadeDrive.vi"("Y axis value"=-0.25 ("X axis value"), "X axis value"=0.5, "RobotDriveDevRef"=w1938) -> ("Motor Values"=w1929:dbl[], "RobotDriveDevRef"=w1939:T16)  [unwired: 1 in, 6 out]
          n466 = call-poly <vilib>:"NT Write Value.vi"("Numeric Array"=w1929, "Name"=w1928) -> ()  [unwired: 9 in, 1 out]
          n467 = call <vilib>:"WPI_RobotDriveDelayAndUpdateSafety.vi"("Delay (s)"=0.5, "RobotDriveDevRef"=w1939) -> ("RobotDriveDevRef 2"=w1940:T16)  [unwired: 8 in, 1 out]
          n468 = call-poly <vilib>:"WPI_RobotDriveArcadeDrive.vi"("Y axis value"=0.0 ("X axis value"), "X axis value"=0.0, "RobotDriveDevRef"=w1940) -> ("Motor Values"=w1930:dbl[])  [unwired: 1 in, 7 out]
          n469 = call-poly <vilib>:"NT Write Value.vi"("Numeric Array"=w1930, "Name"=w1928) -> ()  [unwired: 9 in, 1 out]
        }
        frame "Your Turn" {
          n470 = call <vilib>:"WPI_RobotDriveRefNum Registry Get.vi"("refnum name"="Left and Right Motors") -> ("RobotDriveDevRef"=w1948:T16)  [unwired: 9 in, 1 out]
          n471 = call <vilib>:"WPI_RobotDriveSafetyConfig.vi"("mode"=WPI_SafetyOutputConfigMenu."Disable", "RobotDriveDevRef"=w1948) -> ("RobotDriveDevRef"=w1946:T16)  [unwired: 8 in, 1 out]
          n472 = flat-sequence {
            tunnel: w1946 -> [w1953]
            tunnel: [w1950] -> w1945
            tunnel: w1945 -> [w1956]
            frame #0 {
              w1952 = 1.0
              n473 = Wait (ms)(milliseconds to wait=1000) -> ()  [unwired: 1 out]
              n474 = call-poly <vilib>:"WPI_RobotDriveArcadeDrive.vi"("Y axis value"=w1952, "X axis value"=w1952, "RobotDriveDevRef"=w1953) -> ("RobotDriveDevRef"=w1950:T16)  [unwired: 6 in, 2 out]
            }
            frame #1 {
              w1957 = 0.0
              n475 = call-poly <vilib>:"WPI_RobotDriveArcadeDrive.vi"("Y axis value"=w1957, "X axis value"=w1957, "RobotDriveDevRef"=w1956) -> ("RobotDriveDevRef"=w1955:T16)  [unwired: 6 in, 2 out]
              n476 = Wait (ms)(milliseconds to wait=1000) -> ()  [unwired: 1 out]
              n477 = call <vilib>:"WPI_RobotDriveSafetyConfig.vi"("mode"=WPI_SafetyOutputConfigMenu."Enable", "RobotDriveDevRef"=w1955) -> ()  [unwired: 8 in, 2 out]
            }
          }
        }
        frame "Testing" {
        }
        frame "Low Bar" {
        }
        frame "Portcullis" {
        }
        frame "Cheval" {
        }
        frame "Ramparts" {
        }
        frame "Moat" {
        }
        frame "Drawbridge" {
        }
        frame "Sally Port " {
        }
        frame "Rock Wall" {
        }
        frame "Rough Terrain" {
        }
      }
    }
    frame Enabled {
    }
  }
  n478 = while {
    tunnel: w43 -> [w1967]
    tunnel: w1 -> [w1966]
    stop <- FALSE stop-if-true
    n479 = case shown="\"None\", Default" w1967 {
      tunnel: [120.0 150.0 184.5 160.0 150.0 150.0 120.0 120.0 150.0 150.0 150.0] -> w1960
      frame "None", Default {
      }
      frame "Low Bar" {
      }
      frame "Portcullis" {
      }
      frame "Cheval" {
      }
      frame "Ramparts" {
      }
      frame "Moat" {
      }
      frame "Drawbridge" {
      }
      frame "Sally Port" {
      }
      frame "Rock Wall" {
      }
      frame "Rough Terrain" {
      }
      frame "Test" {
      }
    }
    "Arm Request" <- w1960
    n480 = Wait (ms)(milliseconds to wait=100) -> ()  [unwired: 1 out]
    n481 = call <vilib>:"WPI_MotorControlRefNum Registry Get.vi"("refnum name"="Arm Motor") -> ("MotorControlDevRef"=w1972:T17)  [unwired: 9 in, 1 out]
    n482 = Bundle(w1960, 0.0, FALSE) -> (w1970:cluster{dbl, dbl, bool})  [unwired: 1 in]
    n483 = call "JPL Arm Control EX Autonomous.vi"("Actual Angle"=w1966, "Arm Control"=w1970) -> ("output"=w1959:dbl)  [unwired: 4 in, 1 out]
    "Arm Speed" <- w1959
    n484 = Select(t=w1959, s=FALSE, f=0.0) -> (s? t:f=w1963:dbl)
    n485 = call <vilib>:"WPI_MotorControlSetOutput.vi"("Output"=w1963, "MotorControlDevRef"=w1972) -> ()  [unwired: 7 in, 3 out]
  }
  n486 = call <vilib>:"WPI_RobotDriveRefNum Registry Get.vi"("refnum name"="Left and Right Motors") -> ("RobotDriveDevRef"=w79:T16)  [unwired: 1 in, 9 out]
  n487 = call <vilib>:"WPI_AccelerometerRefNum Registry Get.vi"("refnum name"="AD Accel") -> ("AccelerometerDevRef"=w78:T26)  [unwired: 9 in, 1 out]
  n488 = call <vilib>:"WPI_GyroGetAngle.vi"("GyroDevRef"=w51) -> ("Angle"=→"Vert Gyro Angle":dbl)  [unwired: 6 in, 4 out]
  n489 = call <vilib>:"WPI_GyroGetAngle.vi"("GyroDevRef"=w74) -> ("Angle"=→"Horz Gyro Angle":dbl)  [unwired: 6 in, 4 out]
  n490 = call-poly <vilib>:"NT Read Value.vi"("Name"="Position Selector") -> ("String"=w75:string)  [unwired: 9 in, 1 out]
  "Position" <- w75
  n491 = call <vilib>:"WPI_RelayRefNum Registry Get.vi"("refnum name"="Light Ring") -> ("RelayDevRef"=w7:T32)  [unwired: 9 in, 1 out]
  n492 = call <vilib>:"WPI_ServoRefNum Registry Get.vi"("refnum name"="Camera Servo") -> ("ServoDeviceRef"=w9:T35)  [unwired: 9 in, 1 out]
  n493 = call <vilib>:"WPI_SolenoidRefNum Registry Get.vi"("refnum name"="Retract Catapult") -> ("SolenoidDevRef"=w5:T14)  [unwired: 9 in, 1 out]
  n494 = call <vilib>:"WPI_MotorControlRefNum Registry Get.vi"("refnum name"="Latch") -> ("MotorControlDevRef"=w4:T17)  [unwired: 9 in, 1 out]
